vi "Create control.vi"() -> ()   [LabVIEW 2013]
uses:
  Controls/_ui_tools_font.ctl
  Controls/BX.Orientation__LCR _Modified.ctl
  Typedefs/TypeDef_Action.ctl
  <vilib>/Utility/miscctls.llb/LVPointTypeDef.ctl
  Control.lvclass
  <vilib>/Palette API/Palette Menu/Public Type Define/Palette type.ctl
  <vilib>/Palette API/Palette Menu/Public Type Define/Item.ctl
  Engine/Move Speed.ctl
  <userlib>/_OpenG.lib/array/array.llb/Conditional Auto-Indexing Tunnel (String)__ogtk.vi
  <userlib>/_OpenG.lib/file/file.llb/File Exists - Scalar__ogtk.vi
  <userlib>/_OpenG.lib/file/file.llb/Strip Path - Traditional__ogtk.vi
  <userlib>/_OpenG.lib/file/file.llb/Strip Path Extension - String__ogtk.vi
  <userlib>/_OpenG.lib/string/string.llb/To Proper Case (String)__ogtk.vi
  <vilib>/Utility/config.llb/Read Key (String).vi
  <vilib>/Utility/config.llb/Write Key (String).vi
  Fading/SetTransparency(U8).vi
  Fading/_Fade In(I32).vi
  Fading/_Fade Out(I32).vi
  <vilib>/Utility/config.llb/Read Key (Boolean).vi
  <userlib>/_OpenG.lib/file/file.llb/Build Path - Traditional__ogtk.vi
  <vilib>/Utility/config.llb/NI_LVConfig.lvlib
  <vilib>/Palette API/Palette Menu/Palette Menu.lvlib
panel:
  in  "Same decal True/False":bool
  in  "Tab Control":enum32{"False", "True"}(tab)
  in  "Available Icons":picture[][](array[picture])
  in  "Source directory":path
  in  "Icon source":path
  in  "Toolbar 3":cluster{"Font":T1}={"Font"={"Font Name:"="Tahoma", "Size"=13, "Strikeout?"=FALSE, "Italic?"=FALSE, "Underline?"=FALSE, "Outline?"=FALSE, "Shadow?"=FALSE, "Bold?"=TRUE}}
  in  "Add to Project":bool
  in  "Projects":u16(ring) items=["UI Tools.lvproj"]
  in  "Save *.ctl to disk":bool
  in  "Palette":path=path "_LavaCR/CustomControls" caption="<user.lib>\\"
  in  "Front Panels":u16(ring)
  in  "Drop on Front Panel":bool
  in  "Add a copy to UI Tools Palette":bool
  in  "Cancel":bool
  in  "Create":bool
  in  "TRUE Text":string
  in  "Zoom Min":bool
  in  "Zoom Max":bool
  in  "Scale Icon":dbl(slide)=1.0 min=0.5 max=2.0 scale=0.5..2.0 scale format="%.2g"
  in  "Save for version":u16(ring) items=["13.0", "12.0", "11.0", "10.0", "9.0", "8.6", "8.5", "8.2", "8.0"]
  in  "Action":T2=4 items=["Switch when pressed", "Switch when released", "Switch until release", "Latch when pressed", "Latch when released", "Latch until released"]
  in  "Orientations":T3=14
  in  "Button Style":u16(ring)
  in  "Text Color":u32(colorbox)
  in  "FALSE Text":string
  out "PREVIEW":picture
  # "FONT"
  # "FONT"
  # "Preview"
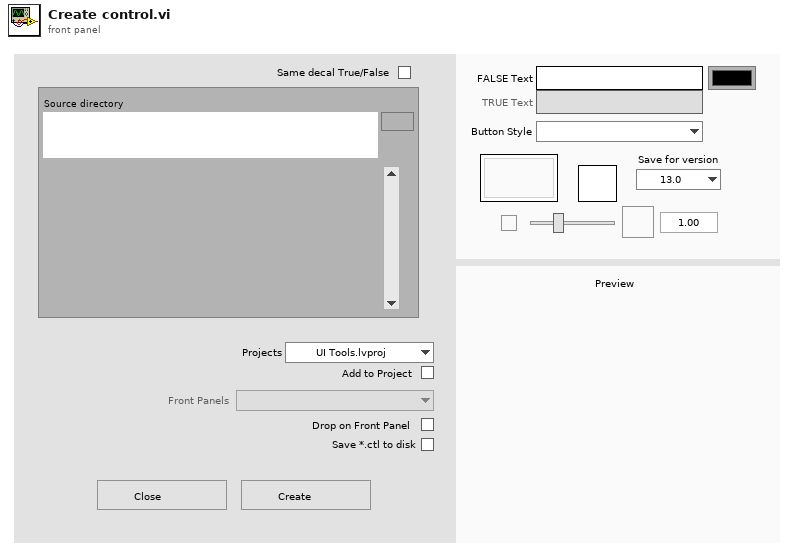
[diagram p1: front panel]
types:
  T1 = typedef "Control.lvclass/_ui_tools_font.ctl" = cluster{"Font Name:":string, "Size":i16, "Strikeout?":bool, "Italic?":bool, "Underline?":bool, "Outline?":bool, "Shadow?":bool, "Bold?":bool}
  T2 = typedef "Control.lvclass/TypeDef_Action.ctl" = u16
  T3 = typedef "Control.lvclass/BX.Orientation__LCR _Modified.ctl" = u8
  T4 = typedef "LVPointTypeDef.ctl" = cluster{"Horizontal":i16, "Vertical":i16}
  T5 = cluster{"Action":refnum<user-event>, "Orientations":refnum<user-event>, "Icon (*.png)":refnum<user-event>, "Font":refnum<user-event>, "Control Text":refnum<user-event>, "Style":refnum<user-event>, "Text Color":refnum<user-event>, "Scale Icon":refnum<user-event>}
  T6 = cluster{"Event Registration Refnum":refnum<event-registration>, "Event Registration Refnum":refnum<event-registration>}
  T7 = typedef "Move Speed.ctl" = enum16{"Normal", "Fast", "Slow", "Instantaneous"}
  T8 = typedef "LVRectTypeDef.ctl" = cluster{"Left":i16, "Top":i16, "Right":i16, "Bottom":i16}
  T9 = cluster{"left":i16, "top":i16, "right":i16, "bottom":i16}
  T10 = cluster{"left":i16, "top":i16, "right":i16, "bottom":i16}[]
  T11 = typedef "LVBoundsTypeDef.ctl" = cluster{"Width":u32, "Height":u32}
  T12 = enum32{"invalid app kind", "Development System", "Run Time System", "Student Edition", "Embedded LabVIEW", "Evaluation", "Custom"}
  T13 = enum32{"Invalid", "Standard", "Closed", "Hidden", "Minimized", "Maximized"}
  T14 = enum32{"Bad", "Idle", "Run top level", "Running"}
  T15 = typedef "Palette Menu.lvlib/Item.ctl" = cluster{"item path":path, "library path (.lvlib)":path, "use default lvlib palette":bool, "short name":string, "place VI contents":bool, "hide synchronized item":bool, "reserve spot for synch item":bool, "configure when placing VI contents":bool}
  T16 = typedef "LVPoint32TypeDef.ctl" = cluster{"Horizontal":i32, "Vertical":i32}
  T17 = typedef "LVPositionTypeDef.ctl" = cluster{"Left":i32, "Top":i32}
  T18 = cluster{"Width":u16, "Style":enum32{"Solid", "Dash", "Dot", "DashDot", "DashDotDot"}}
  T19 = typedef "imagedata.ctl" = cluster{"image type":i32, "image depth":i32, "image":u8[], "mask":u8[], "colors":u32[], "Rectangle":cluster{"left":i16, "top":i16, "right":i16, "bottom":i16}}
  T20 = cluster{"Core":cluster{"Current VI Reference":refnum<vi>, "Close Panel on Exit?":bool, "NI.LV.Dialog namespace":bool, "Menu Launch:App":refnum<vi>, "Local App":refnum<vi>}, "Control":refnum<class "Control.lvclass">, "Errors":cluster{"code":i32, "Short":string, "Long":string, "Critical":bool}[], "user events":cluster{"Action":refnum<user-event>, "Orientations":refnum<user-event>, "Icon (*.png)":refnum<user-event>, "Font":refnum<user-event>, "Control Text":refnum<user-event>, "Style":refnum<user-event>, "Text Color":refnum<user-event>, "Scale Icon":refnum<user-event>}, "last state":cluster{"Action":T2, "Orientations":T3, "Icon (*.png)":path, "Control Text":string, "Style":u16, "Text Color":u32, "Scale":dbl, "Close afterwards":bool}, "config":cluster{"fade":i32, "droplabel":bool}, "file in tmp dir":path, "drop pos":T4}
  T21 = cluster{"code":i32, "Short":string, "Long":string, "Critical":bool}[]
  T22 = cluster{"Action":T2, "Orientations":T3, "Icon (*.png)":path, "Control Text":string, "Style":u16, "Text Color":u32, "Scale":dbl, "Close afterwards":bool}
  T23 = cluster{"Current VI Reference":refnum<vi>, "Close Panel on Exit?":bool, "NI.LV.Dialog namespace":bool, "Menu Launch:App":refnum<vi>, "Local App":refnum<vi>}
  T24 = typedef "NI_LVConfig.lvlib/Config Data RefNum.ctl" = refnum<k1>
  T25 = cluster{"code":i32, "Short":string, "Long":string, "Critical":bool}
  T26 = typedef "Palette Menu.lvlib/Palette type.ctl" = i32
  T27 = typedef "Palette Menu.lvlib/Palette Data.ctl" = cluster{"display name":string, "view format":T28, "palette width":i16, "items":T29, "256 color icon":picture, "B&W color icon":picture, "help information":T30, "palette description":string, "synchronize information":T31}
  T28 = typedef "Palette Menu.lvlib/View Format.ctl" = u16
  T29 = typedef "Palette Menu.lvlib/Items.ctl" = T15[]
  T30 = typedef "Palette Menu.lvlib/Help Info.ctl" = cluster{"help tag":string, "help file path ":path}
  T31 = typedef "Palette Menu.lvlib/Synchronize Info.ctl" = cluster{"synchronize with directory":bool, "synchronize directory path":path}
  T32 = typedef "Control.lvclass/TypeDef_Styles.ctl" = u16
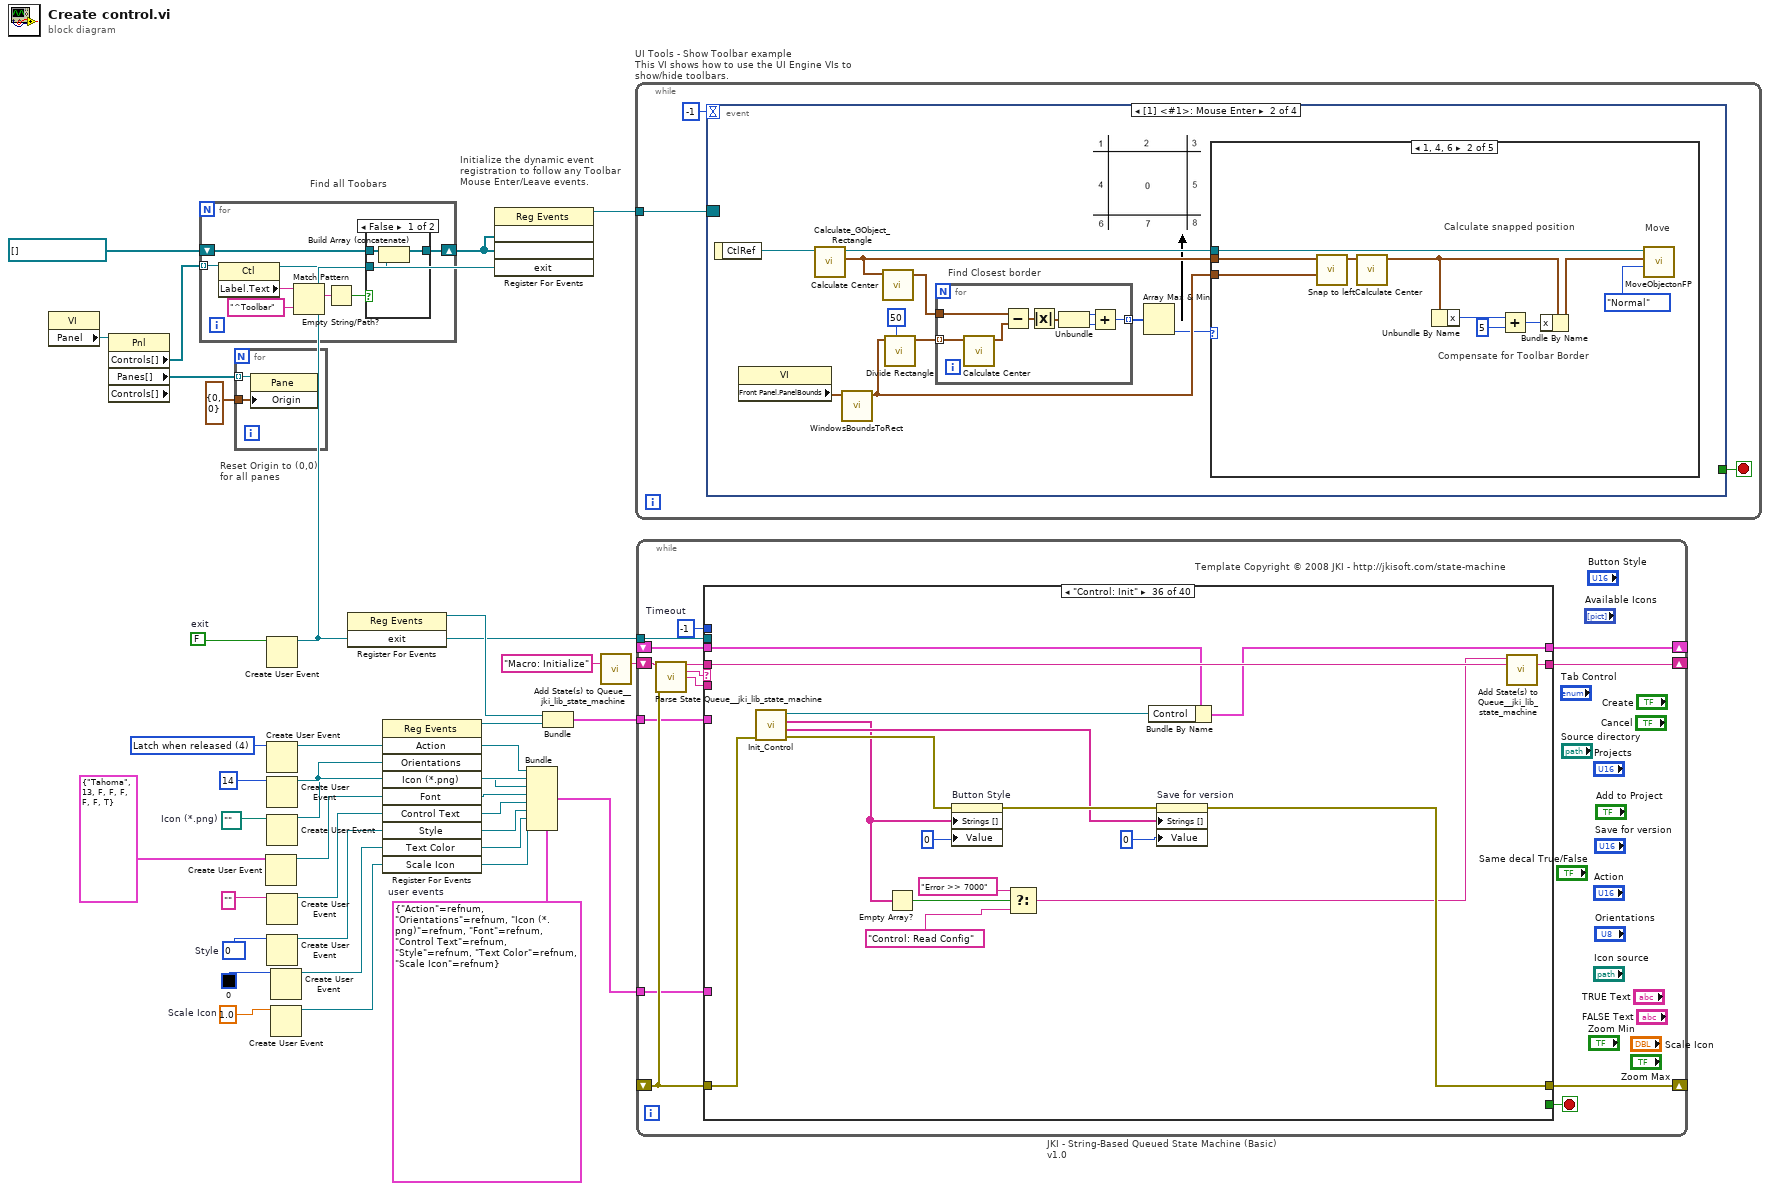
[diagram p0: block diagram]
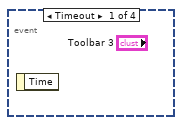
[diagram p3: hidden frame]
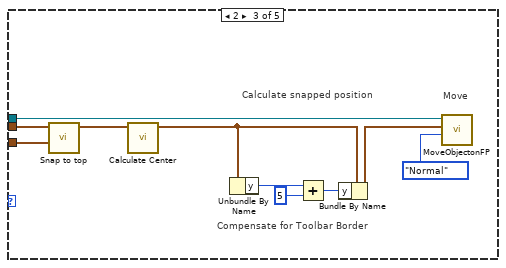
[diagram p5: hidden frame]
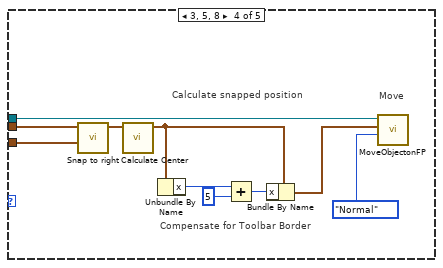
[diagram p6: hidden frame]
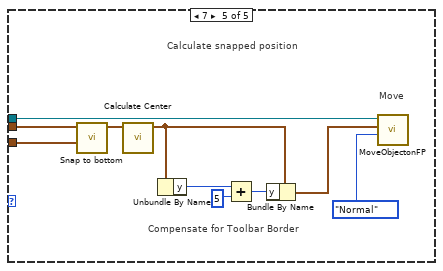
[diagram p7: hidden frame]
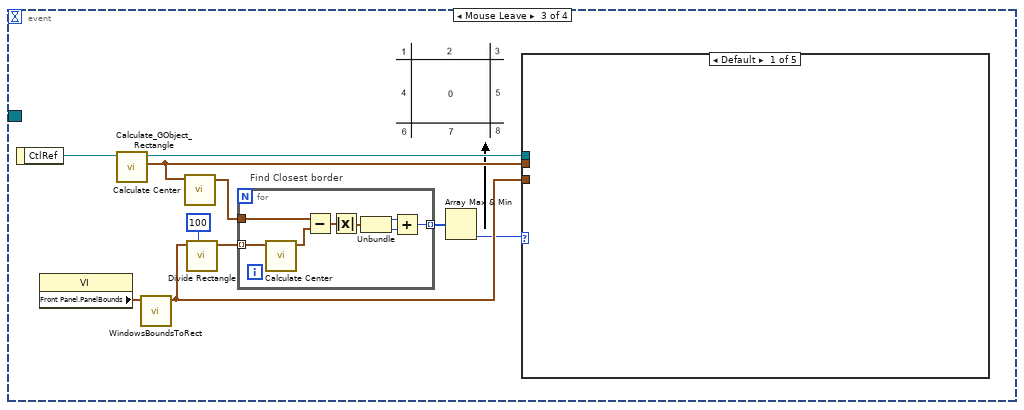
[diagram p8: hidden frame]
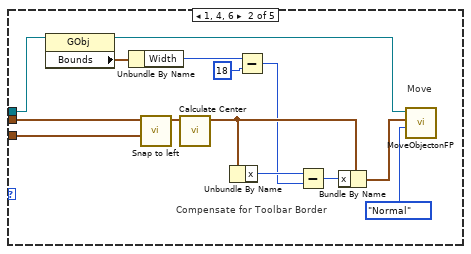
[diagram p9: hidden frame]
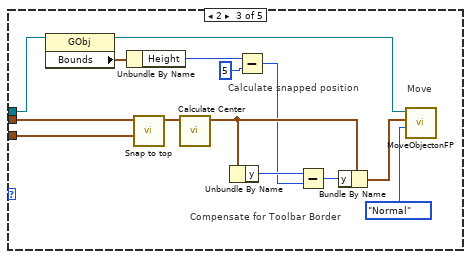
[diagram p10: hidden frame]
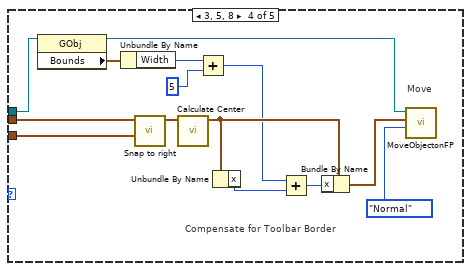
[diagram p11: hidden frame]
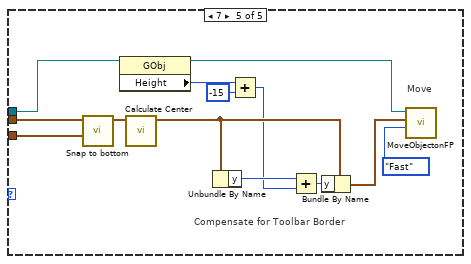
[diagram p12: hidden frame]
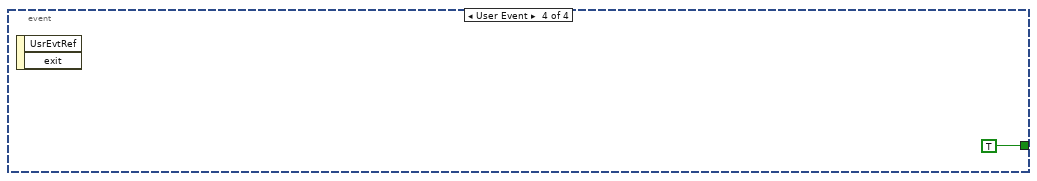
[diagram p13: hidden frame]
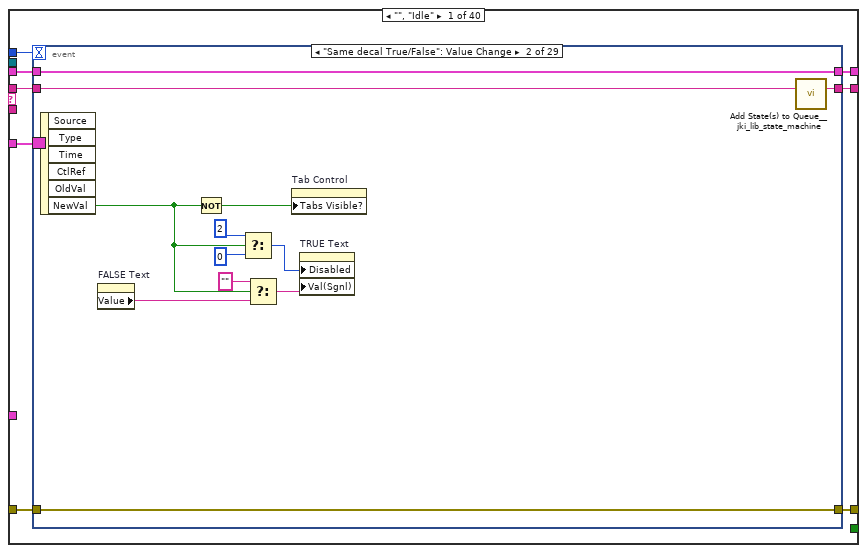
[diagram p14: hidden frame]
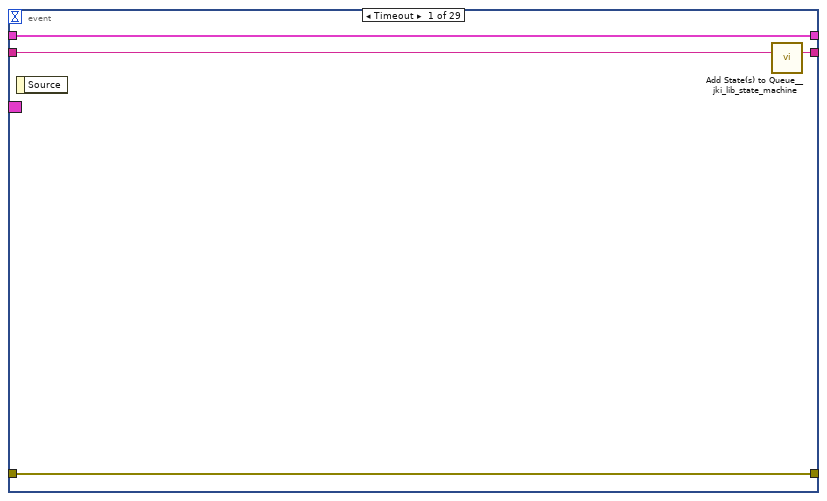
[diagram p15: hidden frame]
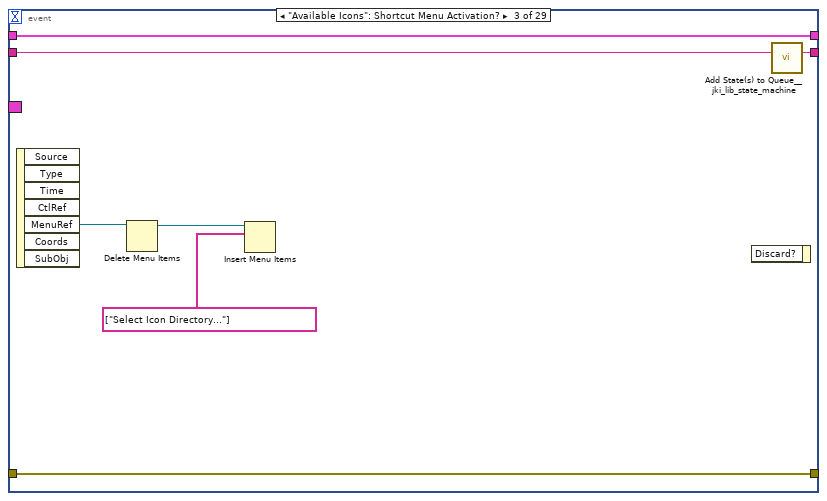
[diagram p16: hidden frame]
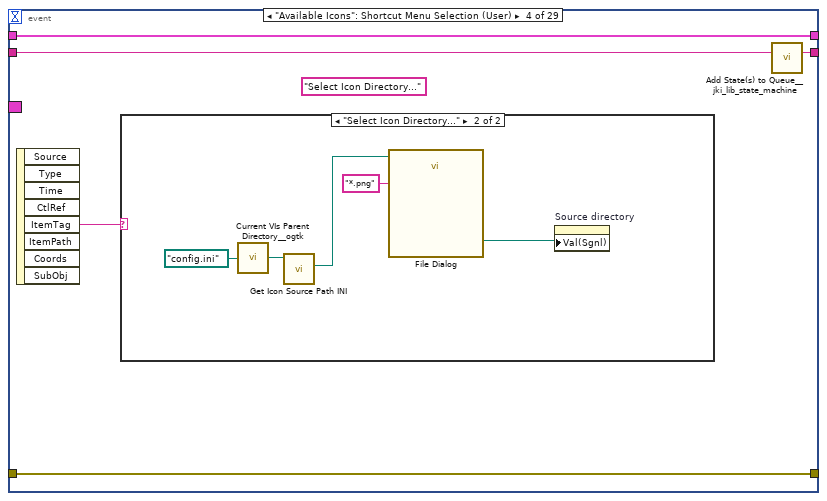
[diagram p17: hidden frame]
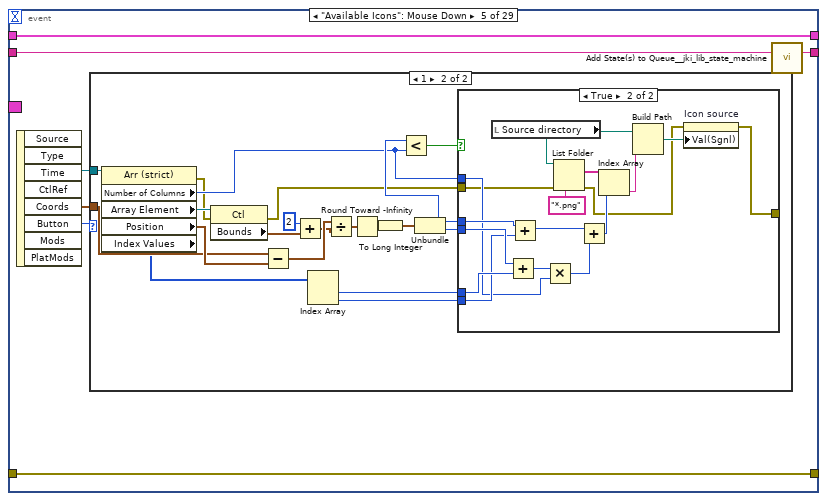
[diagram p19: hidden frame]
diagram:
  w5 = FALSE  # exit
  w13 = T5 {"Action"=refnum, "Orientations"=refnum, "Icon (*.png)"=refnum, "Font"=refnum, "Control Text"=refnum, "Style"=refnum, "Text Color"=refnum, "Scale Icon"=refnum}  # user events
  w18 = 1.0  # Scale Icon
  w22 = u16 0 items=[""]  # Style
  w28 = path ""  # Icon (*.png)
  w32 = T2 4 items=["Switch when pressed", "Switch when released", "Switch until release", "Latch when pressed", "Latch when released", "Latch until released"] ("Action")
  # "Reset Origin to (0,0)\nfor all panes"
  # "Find all Toobars"
  # "Initialize the dynamic event\nregistration to follow any Toolbar\nMouse Enter/Leave events."
  n1 = property class="VI"() -> ("Panel"=w11:refnum<vi>)  [unwired: 2 in, 2 out]
  n2 = property class="Pnl" props=["Controls[]", "Panes[]", "Controls[]"](reference=w11) -> ("Controls[]"=w6:refnum<vi>[], "Panes[]"=w10:refnum<vi>[])  [unwired: 1 in, 3 out]
  n3 = for {
    tunnel: w6 -> [w40] mode=indexing
    shift-right: [w34] -> w7
    shift-left: refnum<vi>[] [] -> [w35]
    n4 = property class="Ctl"(reference=w40) -> (reference out=w33:refnum<vi>, "Label.Text"=w39:string)  [unwired: 1 in, 1 out]
    n5 = Match Pattern(string=w39, regular expression="^Toolbar") -> (match substring=w37:string)  [unwired: 4 out]
    n6 = Empty String/Path?(string/path=w37) -> (empty?=w36:bool)
    n7 = case shown="False" w36 {
      tunnel: [w41 w44] -> w34
      tunnel: w35 -> [w43 w44]
      tunnel: w33 -> [w42 _]
      frame False {
        n8 = Build Array (concatenate)(w43, w42) -> (w41:refnum<vi>[])
      }
      frame True {
      }
    }
  }
  n9 = for {
    tunnel: w10 -> [w46] mode=indexing
    tunnel: T4 {"Horizontal"=0, "Vertical"=0} ("Origin") -> [w45]
    n10 = property class="Pane"(reference=w46, "Origin"=w45) -> ()  [unwired: 1 in, 2 out]
  }
  n11 = Create User Event(user event datatype=T1 {"Font Name:"="Tahoma", "Size"=13, "Strikeout?"=FALSE, "Italic?"=FALSE, "Underline?"=FALSE, "Outline?"=FALSE, "Shadow?"=FALSE, "Bold?"=TRUE} ("Font")) -> (user event=w25:refnum<user-event>)  [unwired: 1 in, 1 out]
  n12 = Create User Event(user event datatype=w5) -> (user event=w1:refnum<user-event>)  [unwired: 1 in, 1 out]
  n13 = Create User Event(user event datatype=w32) -> (user event=w31:refnum<user-event>)  [unwired: 1 in, 1 out]
  n14 = Create User Event(user event datatype=T3 14 ("Orientations")) -> (user event=w30:refnum<user-event>)  [unwired: 1 in, 1 out]
  n15 = Create User Event(user event datatype=w28) -> (user event=w27:refnum<user-event>)  [unwired: 1 in, 1 out]
  n16 = Create User Event(user event datatype="" ("Control Text")) -> (user event=w23:refnum<user-event>)  [unwired: 1 in, 1 out]
  n17 = Create User Event(user event datatype=w22) -> (user event=w21:refnum<user-event>)  [unwired: 1 in, 1 out]
  n18 = Create User Event(user event datatype=u32 0 ("Text Color")) -> (user event=w19:refnum<user-event>)  [unwired: 1 in, 1 out]
  n19 = Create User Event(user event datatype=w18) -> (user event=w17:refnum<user-event>)  [unwired: 1 in, 1 out]
  n20 = register-events(w1) -> (reference out=w4:refnum<event-registration>)  [unwired: 2 in, 1 out]
  n21 = register-events(w31, w30, w27, w25, w23, w21, w19, w17) -> (reference out=w3:refnum<event-registration>)  [unwired: 2 in, 1 out]
  n22 = register-events(w7, w7, w1) -> (reference out=w12:refnum<event-registration>)  [unwired: 2 in, 1 out]
  n23 = Bundle(cluster=w13, "Action"=w31, "Orientations"=w30, "Icon (*.png)"=w27, "Font"=w25, "Control Text"=w23, "Style"=w21, "Text Color"=w19, "Scale Icon"=w17) -> (w14:T5)
  n24 = Bundle("Event Registration Refnum"=w4, "Event Registration Refnum"=w3) -> (w2:T6)  [unwired: 1 out]
  n25 = call <vilib>:"Add State(s) to Queue__jki_lib_state_machine.vi"("State(s) in (\"\")"="Macro: Initialize") -> ("States Out"=w16:string)  [unwired: 2 in, 12 out]
  n26 = while "UI Tools - Show Toolbar example\nThis VI shows how to use the UI Engine VIs to show/hide toolbars." {
    tunnel: w12 -> [w47]
    stop <- w48 stop-if-true
    n27 = event shown="[1] <#1>: Mouse Enter" {
      selector: w47 -> [_ _ _ _]
      dyn-events: _ -> [_ _ _ _]
      timeout: -1 -> [_ _ _ _]
      tunnel: [_ _ _ TRUE ("Discard?")] -> w48
      event Timeout {
        n28 = event-data() -> ()  [unwired: 2 out]
      }
      event Mouse Enter {
        # "Find Closest border"
        n29 = event-data() -> ("CtlRef"=w59:refnum<vi>)  [unwired: 1 out]
        n30 = property class="VI"() -> ("Front Panel.PanelBounds"=w50:T8)  [unwired: 2 in, 2 out]
        n31 = call "Calculate_GObject_Rectangle.vi"("GObject ref"=w59) -> ("Rectangle"=w56:T9, "GObject ref dup"=w51:refnum<vi>)  [unwired: 1 in, 8 out]
        n32 = call "WindowsBoundsToRect.vi"("Windows Bounds"=w50) -> ("Rectangle"=w58:T9)  [unwired: 10 out]
        n33 = call "Calculate Center.vi"("Rectangle"=w56) -> ("Center"=w54:cluster{"x":i32, "y":i32})  [unwired: 10 out]
        n34 = call "Divide Rectangle.vi"("Band (50)"=i16 50, "Rectangle"=w58) -> ("Zones Rectangles"=w55:T10)  [unwired: 1 in, 8 out]
        n35 = for {
          tunnel: w55 -> [w67] mode=indexing
          tunnel: w54 -> [w66]
          tunnel: [w60] -> w53 mode=indexing
          n36 = call "Calculate Center.vi"("Rectangle"=w67) -> ("Center"=w65:cluster{"x":i32, "y":i32})  [unwired: 10 out]
          n37 = Subtract(x=w66, y=w65) -> (x-y=w64:cluster{"x":i32, "y":i32})
          n38 = Absolute Value(x=w64) -> (abs(x)=w63:cluster{"x":i32, "y":i32})
          n39 = Unbundle(w63) -> ("x"=w62:i32, "y"=w61:i32)
          n40 = Add(x=w62, y=w61) -> (x+y=w60:i32)
        }
        n41 = Array Max & Min(array=w53) -> (min index (indices)=w52:i32)  [unwired: 3 out]
        n42 = case shown="1, 4, 6" w52 {
          tunnel: w51 -> [_ w68 w81 w96 w101]
          tunnel: w58 -> [_ w75 w79 w94 w103]
          tunnel: w56 -> [_ w74 w80 w95 w104]
          frame Default {
          }
          frame 1, 4, 6 {
            # "Compensate for Toolbar Border"
            # "Move"
            # "Calculate snapped position"
            n43 = call "Snap to left.vi"("Fixed Rect"=w75, "Rect"=w74) -> ("Snapped to left"=w76:T9)  [unwired: 1 in, 8 out]
            n44 = call "Calculate Center.vi"("Rectangle"=w76) -> ("Center"=w70:cluster{"x":i32, "y":i32})  [unwired: 10 out]
            n45 = Unbundle By Name(w70) -> ("x"=w73:i32)
            n46 = Add(x=w73, y=5) -> (x+y=w71:i32)
            n47 = Bundle By Name(cluster=w70, "x"=w71) -> (w69:cluster{"x":i32, "y":i32})
            n48 = call "MoveObjectonFP.vi"("Move Speed (Instantaneous)"=Move_Speed."Normal", "Center Position for Object"=w69, "GObject"=w68) -> ()  [unwired: 3 in, 6 out]
          }
          frame 2 {
            # "Compensate for Toolbar Border"
            # "Move"
            # "Calculate snapped position"
            n49 = call "Snap to top.vi"("Fixed Rect"=w79, "Rect"=w80) -> ("Snapped to top"=w78:T9)  [unwired: 1 in, 8 out]
            n50 = call "Calculate Center.vi"("Rectangle"=w78) -> ("Center"=w83:cluster{"x":i32, "y":i32})  [unwired: 10 out]
            n51 = Unbundle By Name(w83) -> ("y"=w86:i32)
            n52 = Add(x=w86, y=5) -> (x+y=w84:i32)
            n53 = Bundle By Name(cluster=w83, "y"=w84) -> (w82:cluster{"x":i32, "y":i32})
            n54 = call "MoveObjectonFP.vi"("Move Speed (Instantaneous)"=Move_Speed."Normal", "Center Position for Object"=w82, "GObject"=w81) -> ()  [unwired: 3 in, 6 out]
          }
          frame 3, 5, 8 {
            # "Compensate for Toolbar Border"
            # "Move"
            # "Calculate snapped position"
            n55 = call "Snap to right.vi"("Fixed Rect"=w94, "Rect"=w95) -> ("Snapped to right"=w93:T9)  [unwired: 1 in, 8 out]
            n56 = call "Calculate Center.vi"("Rectangle"=w93) -> ("Center"=w89:cluster{"x":i32, "y":i32})  [unwired: 10 out]
            n57 = Unbundle By Name(w89) -> ("x"=w92:i32)
            n58 = Add(x=w92, y=5) -> (x+y=w90:i32)
            n59 = Bundle By Name(cluster=w89, "x"=w90) -> (w88:cluster{"x":i32, "y":i32})
            n60 = call "MoveObjectonFP.vi"("Move Speed (Instantaneous)"=Move_Speed."Normal", "Center Position for Object"=w88, "GObject"=w96) -> ()  [unwired: 3 in, 6 out]
          }
          frame 7 {
            # "Compensate for Toolbar Border"
            # "Move"
            # "Calculate snapped position"
            n61 = call "Snap to bottom.vi"("Fixed Rect"=w103, "Rect"=w104) -> ("Snapped to bottom"=w102:T9)  [unwired: 1 in, 8 out]
            n62 = call "Calculate Center.vi"("Rectangle"=w102) -> ("Center"=w99:cluster{"x":i32, "y":i32})  [unwired: 10 out]
            n63 = Unbundle By Name(w99) -> ("y"=w106:i32)
            n64 = Add(x=w106, y=5) -> (x+y=w105:i32)
            n65 = Bundle By Name(cluster=w99, "y"=w105) -> (w98:cluster{"x":i32, "y":i32})
            n66 = call "MoveObjectonFP.vi"("Move Speed (Instantaneous)"=Move_Speed."Normal", "Center Position for Object"=w98, "GObject"=w101) -> ()  [unwired: 3 in, 6 out]
          }
        }
      }
      event Mouse Leave {
        # "Find Closest border"
        n67 = event-data() -> ("CtlRef"=w110:refnum<vi>)  [unwired: 1 out]
        n68 = property class="VI"() -> ("Front Panel.PanelBounds"=w109:T8)  [unwired: 2 in, 2 out]
        n69 = call "Calculate_GObject_Rectangle.vi"("GObject ref"=w110) -> ("Rectangle"=w114:T9, "GObject ref dup"=w117:refnum<vi>)  [unwired: 1 in, 8 out]
        n70 = call "WindowsBoundsToRect.vi"("Windows Bounds"=w109) -> ("Rectangle"=w116:T9)  [unwired: 10 out]
        n71 = call "Calculate Center.vi"("Rectangle"=w114) -> ("Center"=w112:cluster{"x":i32, "y":i32})  [unwired: 10 out]
        n72 = call "Divide Rectangle.vi"("Band (50)"=i16 100, "Rectangle"=w116) -> ("Zones Rectangles"=w113:T10)  [unwired: 1 in, 8 out]
        n73 = for {
          tunnel: w113 -> [w125] mode=indexing
          tunnel: w112 -> [w124]
          tunnel: [w118] -> w111 mode=indexing
          n74 = call "Calculate Center.vi"("Rectangle"=w125) -> ("Center"=w123:cluster{"x":i32, "y":i32})  [unwired: 10 out]
          n75 = Subtract(x=w124, y=w123) -> (x-y=w122:cluster{"x":i32, "y":i32})
          n76 = Absolute Value(x=w122) -> (abs(x)=w121:cluster{"x":i32, "y":i32})
          n77 = Unbundle(w121) -> ("x"=w120:i32, "y"=w119:i32)
          n78 = Add(x=w120, y=w119) -> (x+y=w118:i32)
        }
        n79 = Array Max & Min(array=w111) -> (min index (indices)=w108:i32)  [unwired: 3 out]
        n80 = case shown="Default" w108 {
          tunnel: w117 -> [_ w130 w147 w160 w172]
          tunnel: w116 -> [_ w137 w141 w165 w176]
          tunnel: w114 -> [_ w136 w142 w166 w177]
          frame Default {
          }
          frame 1, 4, 6 {
            # "Compensate for Toolbar Border"
            # "Move"
            n81 = property class="GObj"(reference=w130) -> (reference out=w129:refnum<vi>, "Bounds"=w131:T11)  [unwired: 1 in, 1 out]
            n82 = Unbundle By Name(w131) -> ("Width"=w128:u32)
            n83 = call "Snap to left.vi"("Fixed Rect"=w137, "Rect"=w136) -> ("Snapped to left"=w138:T9)  [unwired: 1 in, 8 out]
            n84 = call "Calculate Center.vi"("Rectangle"=w138) -> ("Center"=w133:cluster{"x":i32, "y":i32})  [unwired: 10 out]
            n85 = Unbundle By Name(w133) -> ("x"=w135:i32)
            n86 = Subtract(x=w128, y=u32 18) -> (x-y=w126:u32)
            n87 = Subtract(x=w135, y=w126) -> (x-y=w134:u32)
            n88 = Bundle By Name(cluster=w133, "x"=w134) -> (w132:cluster{"x":i32, "y":i32})
            n89 = call "MoveObjectonFP.vi"("Move Speed (Instantaneous)"=Move_Speed."Normal", "Center Position for Object"=w132, "GObject"=w129) -> ()  [unwired: 3 in, 6 out]
          }
          frame 2 {
            # "Compensate for Toolbar Border"
            # "Move"
            # "Calculate snapped position"
            n90 = property class="GObj"(reference=w147) -> (reference out=w146:refnum<vi>, "Bounds"=w148:T11)  [unwired: 1 in, 1 out]
            n91 = Unbundle By Name(w148) -> ("Height"=w145:u32)
            n92 = call "Snap to top.vi"("Fixed Rect"=w141, "Rect"=w142) -> ("Snapped to top"=w140:T9)  [unwired: 1 in, 8 out]
            n93 = call "Calculate Center.vi"("Rectangle"=w140) -> ("Center"=w150:cluster{"x":i32, "y":i32})  [unwired: 10 out]
            n94 = Unbundle By Name(w150) -> ("y"=w152:i32)
            n95 = Subtract(x=w145, y=u32 5) -> (x-y=w143:u32)
            n96 = Subtract(x=w152, y=w143) -> (x-y=w151:u32)
            n97 = Bundle By Name(cluster=w150, "y"=w151) -> (w149:cluster{"x":i32, "y":i32})
            n98 = call "MoveObjectonFP.vi"("Move Speed (Instantaneous)"=Move_Speed."Normal", "Center Position for Object"=w149, "GObject"=w146) -> ()  [unwired: 3 in, 6 out]
          }
          frame 3, 5, 8 {
            # "Compensate for Toolbar Border"
            # "Move"
            n99 = property class="GObj"(reference=w160) -> (reference out=w159:refnum<vi>, "Bounds"=w161:T11)  [unwired: 1 in, 1 out]
            n100 = Unbundle By Name(w161) -> ("Width"=w156:u32)
            n101 = call "Snap to right.vi"("Fixed Rect"=w165, "Rect"=w166) -> ("Snapped to right"=w164:T9)  [unwired: 1 in, 8 out]
            n102 = call "Calculate Center.vi"("Rectangle"=w164) -> ("Center"=w163:cluster{"x":i32, "y":i32})  [unwired: 10 out]
            n103 = Add(x=w156, y=5) -> (x+y=w154:u32)
            n104 = Unbundle By Name(w163) -> ("x"=w158:i32)
            n105 = Add(x=w154, y=w158) -> (x+y=w157:u32)
            n106 = Bundle By Name(cluster=w163, "x"=w157) -> (w162:cluster{"x":i32, "y":i32})
            n107 = call "MoveObjectonFP.vi"("Move Speed (Instantaneous)"=Move_Speed."Normal", "Center Position for Object"=w162, "GObject"=w159) -> ()  [unwired: 3 in, 6 out]
          }
          frame 7 {
            # "Compensate for Toolbar Border"
            # "Move"
            n108 = call "Snap to bottom.vi"("Fixed Rect"=w176, "Rect"=w177) -> ("Snapped to bottom"=w175:T9)  [unwired: 1 in, 8 out]
            n109 = property class="GObj"(reference=w172) -> (reference out=w171:refnum<vi>, "Height"=w174:u32)  [unwired: 1 in, 1 out]
            n110 = call "Calculate Center.vi"("Rectangle"=w175) -> ("Center"=w179:cluster{"x":i32, "y":i32})  [unwired: 10 out]
            n111 = Unbundle By Name(w179) -> ("y"=w169:i32)
            n112 = Add(x=w174, y=-15) -> (x+y=w168:u32)
            n113 = Add(x=w169, y=w168) -> (x+y=w170:u32)
            n114 = Bundle By Name(cluster=w179, "y"=w170) -> (w178:cluster{"x":i32, "y":i32})
            n115 = call "MoveObjectonFP.vi"("Move Speed (Instantaneous)"=Move_Speed."Fast", "Center Position for Object"=w178, "GObject"=w171) -> ()  [unwired: 3 in, 6 out]
          }
        }
      }
      event User Event {
        n116 = event-data() -> ()  [unwired: 3 out]
      }
    }
  }
  n117 = while "JKI - String-Based Queued State Machine (Basic) v1.0" {
    shift-right: [w188] -> _
    shift-left: _ -> [w187]
    shift-right: [w191] -> _
    shift-left: _ -> [w185]
    shift-right: [w190] -> _
    shift-left: w16 -> [w192]
    tunnel: w14 -> [w184]
    tunnel: w2 -> [w183]
    tunnel: w1 -> [w182]
    stop <- w189 stop-if-true
    w186 = -1  # Timeout
    # "Template Copyright © 2008 JKI - http://jkisoft.com/state-machine"
    n118 = call <vilib>:"Parse State Queue__jki_lib_state_machine.vi"("State Queue"=w192, "Error In (no error)"=w185) -> ("Remaining States"=w194:string, "Current State"=w195:string, "Arguments"=w193:string)  [unwired: 11 out]
    n119 = case shown="\"Control: Init\"" w195 {
      selector: w195 -> [_ _ w613 _ _ _ _ _ _ _ _ _ _ _ _ _ _ _ _ _ _ _ _ _ _ _ _ _ _ _ _ _ _ _ _ _ _ _ _ _]
      tunnel: w194 -> [w203 w612 w617 w627 w645 w655 w680 w692 w696 w708 w732 w745 w756 w775 w789 w796 w802 w805 w814 w859 w880 w903 w908 w919 w923 w943 w967 w996 w1036 w1044 w1067 w1117 w1149 w1191 w1211 w1228 w1240 w1292 w1328 w1360]
      tunnel: w193 -> [_ _ _ _ _ _ w678 _ _ _ _ _ _ _ w785 _ _ w806 w816 _ _ _ _ _ _ _ _ _ _ _ _ _ _ _ _ _ _ _ _ _]
      tunnel: w187 -> [w201 w609 w615 w624 w636 w652 w677 w690 w693 _ w728 w742 w748 w759 w787 w794 w803 w809 w818 w845 w867 w900 w905 w911 w920 w941 w952 w981 w1033 w1041 w1065 w1099 w1147 w1151 w1208 w1226 w1241 w1290 w1335 w1347]
      tunnel: [w200 w610 w619 w625 w642 errorcluster {"status"=FALSE, "code"=0, "source"=""} ("error out") w674 w689 w694 w705 w718 w743 w746 w761 w780 w790 w797 w807 w819 w857 w878 w901 w906 w909 w921 w928 w944 w994 w1034 w1042 w1049 w1107 w1139 w1164 w1209 w1218 w1246 w1294 w1315 w1341] -> w191
      tunnel: w185 -> [w199 w610 w618 w625 w642 w647 _ w689 w694 w705 w729 w743 w746 w762 w781 w791 w798 w808 w820 w857 w878 w901 w906 w909 w921 w931 w947 w994 w1034 w1042 w1048 w1106 w1140 w1169 w1209 w1219 w1247 w1295 w1314 w1342]
      tunnel: [w202 w611 w616 w626 w644 w654 w679 w691 w695 w707 w731 w744 w755 w774 w788 w795 w801 w804 w815 w858 w879 w902 w907 w918 w922 w942 w966 w995 w1035 w1043 w1066 w1116 w1148 w1190 w1210 w1227 w1244 w1293 w1326 w1359] -> w190
      tunnel: [_ _ _ _ _ _ _ TRUE _ _ _ _ _ _ _ _ _ _ _ _ _ _ _ _ _ _ _ _ _ _ _ _ _ _ _ _ _ _ _ _] -> w189
      tunnel: [w198 w609 w615 w624 w643 w652 w677 w690 w693 w706 w728 w742 w748 w758 w787 w794 w803 w809 w818 w845 w867 w900 w905 w911 w920 w941 w951 w980 w1032 w1040 w1064 w1115 w1146 w1189 w1207 w1225 w1237 w1291 w1335 w1346] -> w188
      tunnel: w186 -> [w197 _ _ _ _ _ _ _ _ _ _ _ _ _ _ _ _ _ _ _ _ _ _ _ _ _ _ _ _ _ _ _ _ _ _ _ _ _ _ _]
      tunnel: w184 -> [_ _ _ _ _ _ _ _ _ w701 _ _ _ _ _ _ _ _ _ _ _ _ _ _ _ _ _ _ _ _ _ _ _ _ _ _ _ _ _ _]
      tunnel: w183 -> [w196 _ _ _ _ _ _ _ _ _ w711 _ _ _ _ _ _ _ _ _ _ _ _ _ _ _ _ _ _ _ _ _ _ _ _ _ _ _ _ _]
      tunnel: w182 -> [_ _ _ _ _ _ _ w687 _ _ _ _ _ _ _ _ _ _ _ _ _ _ _ _ _ _ _ _ _ _ _ _ _ _ _ _ _ _ _ _]
      frame "", "Idle" {
        # "executes when the state queue is empty"
        n120 = event shown="[1] \"Same decal True/False\": Value Change" {
          selector: w196 -> [_ _ _ _ _ _ _ _ _ _ _ _ _ _ _ _ _ _ _ _ _ _ _ _ _ _ _ _ _]
          dyn-events: _ -> [_ _ _ _ _ _ _ _ _ _ _ _ _ _ _ _ _ _ _ _ _ _ _ _ _ _ _ _ _]
          timeout: w197 -> [_ _ _ _ _ _ _ _ _ _ _ _ _ _ _ _ _ _ _ _ _ _ _ _ _ _ _ _ _]
          tunnel: w203 -> [w207 w219 w226 w231 w243 w314 w323 w359 w365 w376 w386 w396 w409 w419 w429 w439 w451 w473 w497 w508 w518 w528 w541 w551 w561 w582 w592 w602 w604]
          tunnel: [w206 w218 w225 w230 w242 w313 w322 w358 w364 w375 w385 w395 w408 w418 w428 w438 w450 w472 w496 w507 w517 w527 w540 w550 w560 w581 w591 w601 w603] -> w202
          tunnel: w201 -> [w204 w216 w223 w228 w240 w311 w350 w356 w362 w373 w383 w393 w406 w416 w426 w436 w448 w470 w494 w505 w515 w525 w538 w548 w558 w579 w589 w599 w607]
          tunnel: [w205 w217 w224 w229 w241 w312 w351 w357 w363 w367 w377 w387 w401 w410 w420 w430 w440 w463 w491 w502 w512 w522 w535 w545 w555 w570 w583 w593 w608] -> w200
          tunnel: w199 -> [w205 w217 w224 w229 w241 w312 w351 w357 w363 w368 w378 w388 w402 w411 w421 w431 w441 w462 w487 w499 w510 w520 w533 w543 w553 w572 w584 w594 w608]
          tunnel: [w204 w216 w223 w228 w240 w311 w350 w356 w362 w372 w382 w392 w405 w415 w425 w435 w447 w469 w493 w504 w514 w524 w537 w547 w557 w578 w588 w598 w607] -> w198
          event Timeout {
            n121 = event-data() -> ()  [unwired: 2 out]
            n122 = call <vilib>:"Add State(s) to Queue__jki_lib_state_machine.vi"("State(s) in (\"\")"=w207) -> ("States Out"=w206:string)  [unwired: 2 in, 12 out]
          }
          event "Same decal True/False": Value Change {
            n123 = event-data() -> ("NewVal"=w210:bool)  [unwired: 6 out]
            n124 = property on="FALSE Text" class="Str"() -> ("Value"=w209:string)  [unwired: 2 in, 2 out]
            n125 = Not(x=w210) -> (.not. x?=w215:bool)
            n126 = Select(t=u8 2 ("Disabled"), s=w210, f=u8 0 ("Disabled")) -> (s? t:f=w212:u8)
            n127 = Select(t="", s=w210, f=w209) -> (s? t:f=w211:string)
            n128 = property on="Tab Control" class="TabCtl (strict)"("Tabs Visible?"=w215) -> ()  [unwired: 2 in, 2 out]
            n129 = property on="TRUE Text" class="Str"("Disabled"=w212, "Val(Sgnl)"=w211) -> ()  [unwired: 2 in, 2 out]
            n130 = call <vilib>:"Add State(s) to Queue__jki_lib_state_machine.vi"("State(s) in (\"\")"=w219) -> ("States Out"=w218:string)  [unwired: 2 in, 12 out]
          }
          event "Available Icons": Shortcut Menu Activation? {
            n131 = event-data() -> ("MenuRef"=w222:refnum<k9>)  [unwired: 7 out]
            n132 = Delete Menu Items(9:w222) -> (3:w221:refnum<k9>)  [unwired: 1 in, 3 out]
            n133 = Insert Menu Items(8:string[] ["Select Icon Directory..."] ("item names"), 9:w221) -> ()  [unwired: 1 in, 6 out]
            n134 = event-data() -> ()  [unwired: 1 in, 2 out]
            n135 = call <vilib>:"Add State(s) to Queue__jki_lib_state_machine.vi"("State(s) in (\"\")"=w226) -> ("States Out"=w225:string)  [unwired: 2 in, 12 out]
          }
          event "Available Icons": Shortcut Menu Selection (User) {
            (unwired) "Select Icon Directory..."
            n136 = event-data() -> ("ItemTag"=w227:string)  [unwired: 8 out]
            n137 = case shown="\"Select Icon Directory...\"" w227 {
              frame "False", Default {
              }
              frame "Select Icon Directory..." {
                n138 = call <userlib>:"Current VIs Parent Directory__ogtk.vi"("Relative path (.)"=path "config.ini") -> ("Parent Directory (+ Relative)"=w234:path)  [unwired: 4 out]
                n139 = call "Get Icon Source Path INI.vi"("config.ini path"=w234) -> ("Icon source dir"=w232:path)  [unwired: 2 in, 8 out]
                n140 = call "File Dialog"("start path"=w232, "pattern (all files)"="*.png") -> ("selected path"=w233:path)  [unwired: 5 in, 8 out]
                n141 = property on="Source directory" class="Path"("Val(Sgnl)"=w233) -> ()  [unwired: 2 in, 2 out]
              }
            }
            n142 = call <vilib>:"Add State(s) to Queue__jki_lib_state_machine.vi"("State(s) in (\"\")"=w231) -> ("States Out"=w230:string)  [unwired: 2 in, 12 out]
          }
          event "Available Icons": Mouse Down {
            n143 = event-data() -> ("CtlRef"=w239:refnum<vi>, "Coords"=w238:T16, "Button"=w237:u16)  [unwired: 6 out]
            n144 = case shown="1" w237 {
              tunnel: w239 -> [_ w263]
              tunnel: w238 -> [_ w260]
              frame Default {
              }
              frame 1 {
                n145 = property class="Arr (strict)"(reference=w263) -> (error out=w245:errorcluster, "Number of Columns"=w246:u32, "Array Element"=w262:refnum<vi>, "Position"=w261:T17, "Index Values"=w255:u32[])  [unwired: 1 in, 1 out]
                n146 = property class="Ctl"(reference=w262, error in=w245) -> (error out=w244:errorcluster, "Bounds"=w251:T11)  [unwired: 1 out]
                n147 = Subtract(x=w260, y=w261) -> (x-y=w259:T16)
                n148 = Add(x=2, y=w251) -> (x+y=w250:T11)
                n149 = Index Array(array=w255) -> (element #1=w253:u32, element #2=w252:u32)  [unwired: 2 in]
                n150 = Divide(x=w259, y=w250) -> (x/y=w258:cluster{dbl, dbl})
                n151 = Round Toward -Infinity(1:w258) -> (0:w257:cluster{dbl, dbl})
                n152 = To Long Integer(number=w257) -> (32bit integer=w256:cluster{i32, i32})
                n153 = Unbundle(w256) -> (w247:i32, w254:i32)
                n154 = Less?(x=w247, y=w246) -> (x < y?=w248:bool)
                n155 = case shown="True" w248 {
                  tunnel: w247 -> [_ w280]
                  tunnel: w254 -> [_ w279]
                  tunnel: w253 -> [_ w269]
                  tunnel: w252 -> [_ w268]
                  tunnel: w246 -> [_ w267]
                  tunnel: [_ w265] -> _
                  tunnel: w244 -> [_ w264]
                  frame False {
                  }
                  frame True {
                    n156 = local read "Source directory"() -> (w272:path)
                    n157 = Add(x=w279, y=w269) -> (x+y=w275:u32)
                    n158 = Add(x=w280, y=w268) -> (x+y=w273:u32)
                    n159 = Multiply(x=w275, y=w267) -> (x*y=w274:u32)
                    n160 = List Folder(path=w272, pattern="*.png", error in=w264) -> (filenames=w277:string[], error out=w266:errorcluster)  [unwired: 3 out]
                    n161 = Add(x=w273, y=w274) -> (x+y=w276:u32)
                    n162 = Index Array(array=w277, index=w276) -> (element=w271:string)
                    n163 = Build Path(base path=w272, name or relative path=w271) -> (appended path=w270:path)
                    n164 = property on="Icon source" class="Path"(error in=w266, "Val(Sgnl)"=w270) -> (error out=w265:errorcluster)  [unwired: 1 in, 1 out]
                  }
                }
              }
            }
            n165 = call <vilib>:"Add State(s) to Queue__jki_lib_state_machine.vi"("State(s) in (\"\")"=w243) -> ("States Out"=w242:string)  [unwired: 2 in, 12 out]
          }
          event "Source directory": Value Change {
            w292 = T18 {"Width"=2, "Style"=enum."Dash"} ("pen")
            w288 = i16 4 ("oval width")
            n166 = event-data() -> ("NewVal"=w282:path)  [unwired: 1 out]
            n167 = property on="Icon source" class="Path"() -> ("Value"=w305:path)  [unwired: 2 in, 2 out]
            n168 = Strip Path(path=w305) -> (name=w303:string)  [unwired: 1 out]
            n169 = List Folder(path=w282, pattern="*.png") -> (path out=w309:path, filenames=w304:string[], error out=w283:errorcluster)  [unwired: 1 in, 2 out]
            n170 = property on="Available Icons" class="Arr (strict)"() -> ("Number of Columns"=w294:u32, "Array Element"=w293:refnum<vi>)  [unwired: 2 in, 2 out]
            n171 = Search 1D Array(1D array=w304, element=w303) -> (index of element=w302:i32)  [unwired: 1 out]
            n172 = for {
              tunnel: w304 -> [w318] mode=indexing
              tunnel: w309 -> [w319]
              tunnel: [w315] -> w308 mode=indexing
              tunnel: w283 -> [_]
              n173 = Build Path(base path=w319, name or relative path=w318) -> (appended path=w317:path)
              n174 = call <vilib>:"Read PNG File.vi"("path to PNG file"=w317) -> ("image data"=w316:T19)  [unwired: 1 in, 9 out]
              n175 = call <vilib>:"Draw Flattened Pixmap.vi"("image data"=w316) -> ("new picture"=w315:picture)  [unwired: 1 in, 7 out]
            }
            n176 = property class="Ctl"(reference=w293) -> ("Bounds"=w291:T11)  [unwired: 1 in, 2 out]
            n177 = Unbundle By Name(w292) -> ("Width"=w290:u16)
            n178 = Array Size(array=w308) -> (size(s)=w307:i32)
            n179 = Subtract(x=w291, y=w290) -> (x-y=w289:T11)
            n180 = Quotient & Remainder(x=w302, y=w294) -> (x-y*floor(x/y)=w295:u32, floor(x/y)=w296:u32)
            n181 = Quotient & Remainder(x=w307, y=w294) -> (floor(x/y)=w306:u32)  [unwired: 1 out]
            n182 = Reshape Array(w308, w306, w294) -> (w301:picture[][])
            n183 = Index Array(array=w301, index (row)=w296, index (col)=w295) -> (element=w299:picture)
            n184 = Subtract(x=w289, y=w288) -> (x-y=w287:T11)
            n185 = Unbundle(w287) -> ("Width"=w281:u32, "Height"=w284:u32)
            n186 = Bundle(cluster=T9 {"left"=0, "top"=0, "right"=42, "bottom"=42} ("rect"), "right"=w281, "bottom"=w284) -> (w285:T9)  [unwired: 2 out]
            n187 = call <vilib>:"Draw Round Rect.vi"("picture"=w299, "oval width"=w288, "rect"=w285, "color(black)"=u32 35073, "oval height"=w288, "pen"=w292) -> ("new picture"=w298:picture)  [unwired: 1 in, 2 out]
            n188 = Replace Array Subset(array=w301, new element=w298, index (row)=w296, index (col)=w295) -> (w300:picture[][])
            n189 = property on="Available Icons" class="Arr (strict)"("Value"=w300) -> ()  [unwired: 2 in, 2 out]
            n190 = call <vilib>:"Add State(s) to Queue__jki_lib_state_machine.vi"("State(s) in (\"\")"=w314) -> ("States Out"=w313:string)  [unwired: 2 in, 12 out]
          }
          event "Create": Value Change {
            # "If batch processing needed, prepare for it."
            # "Prepare for the execution list based on\nuser choices."
            n191 = event-data() -> ()  [unwired: 2 out]
            n192 = property on="Add to Project" class="Bool (strict)"() -> ("Value"=w321:bool)  [unwired: 2 in, 2 out]
            n193 = property on="Icon source" class="Path"() -> ("Value"=w320:path)  [unwired: 2 in, 2 out]
            n194 = call-poly <userlib>:"File Exists__ogtk.vi"("file path"=w320) -> ("is directory"=w338:bool, "exists"=w337:bool)  [unwired: 6 in]
            n195 = And(x=w338, y=w337) -> (x .and. y?=w335:bool)
            n196 = Build Array("Save *.ctl to disk", "Add a copy to UI Tools Palette", w321, "Drop on Front Panel") -> (w342:bool[])
            n197 = Build Array("Control: Save Control to Disk", "Control: Add to palette", "Control: Add to Project", "Control: Add to FP") -> (w341:string[])
            n198 = call-poly <userlib>:"Conditional Auto-Indexing Tunnel__ogtk.vi"("Array in"=w341, "Elements to keep"=w342) -> ("Filtered Array out"=w340:string[])  [unwired: 5 out]
            n199 = for {
              tunnel: w340 -> [w354] mode=indexing
              shift-right: [w352] -> w326
              shift-left: "" -> [w353]
              n200 = call <vilib>:"Add State(s) to Queue__jki_lib_state_machine.vi"("State(s) in (\"\")"=w353, "State(s) at Back (\"\")"=w354) -> ("States Out"=w352:string)  [unwired: 1 in, 12 out]
            }
            n201 = Select(t="Control: Prepare batch", s=w335, f="") -> (s? t:f=w329:string)
            n202 = Select(t="Macro: Exit", s=FALSE ("End program afterwards"), f="") -> (s? t:f=w328:string)
            n203 = call <vilib>:"Add State(s) to Queue__jki_lib_state_machine.vi"("State(s) in Front (\"\")"="Control: Save Temp Control", "State(s) in (\"\")"=w326, "State(s) at Back (\"\")"="Control: Save Config\nControl: Delete Temp Control") -> ("States Out"=w330:string)  [unwired: 12 out]
            n204 = call <vilib>:"Add State(s) to Queue__jki_lib_state_machine.vi"("State(s) in Front (\"\")"=w329, "State(s) in (\"\")"=w330, "State(s) at Back (\"\")"=w328) -> ("States Out"=w324:string)  [unwired: 12 out]
            n205 = call <vilib>:"Add State(s) to Queue__jki_lib_state_machine.vi"("State(s) in Front (\"\")"=w324, "State(s) in (\"\")"=w323) -> ("States Out"=w322:string)  [unwired: 1 in, 12 out]
          }
          event "Cancel": Value Change {
            # "Exit Button Value Change (pressed) Event\n(this executes Macro: Exit to terminate the VI)"
            n206 = event-data() -> ()  [unwired: 2 out]
            n207 = call <vilib>:"Add State(s) to Queue__jki_lib_state_machine.vi"("State(s) in Front (\"\")"="Macro: Exit", "State(s) in (\"\")"=w359) -> ("States Out"=w358:string)  [unwired: 1 in, 12 out]
          }
          event Menu Selection (User) {
            # "Menu selections (including rtm file)"
            n208 = event-data() -> ("ItemTag"=w360:string)  [unwired: 7 out]
            n209 = case shown="\"About\"" w360 {
              tunnel: [_ "UI: FadeOut >> 200\nAbout\nUI: FadeIn >> 200"] -> w361
              frame Default {
              }
              frame "About" {
              }
            }
            n210 = call <vilib>:"Add State(s) to Queue__jki_lib_state_machine.vi"("State(s) in Front (\"\")"=w361, "State(s) in (\"\")"=w365) -> ("States Out"=w364:string)  [unwired: 1 in, 12 out]
          }
          event Value Change {
            n211 = event-data() -> ("NewVal"=w369:T1)  [unwired: 6 out]
            n212 = Unbundle By Name(w373) -> ("Control"=w371:refnum<class "Control.lvclass">)
            n213 = call-dynamic "Write Text Font.vi"("error in (no error)"=w368, "Font"=w369, "Control in"=w371) -> ("error out"=w367:errorcluster, "Control out"=w370:refnum<class "Control.lvclass">)  [unwired: 7 out]
            n214 = Bundle By Name(cluster=w373, "Control"=w370) -> (w372:T20)
            n215 = call <vilib>:"Add State(s) to Queue__jki_lib_state_machine.vi"("State(s) in Front (\"\")"="Preview", "State(s) in (\"\")"=w376) -> ("States Out"=w375:string)  [unwired: 1 in, 12 out]
          }
          event "Scale Icon": Value Change {
            n216 = event-data() -> ("NewVal"=w379:dbl)  [unwired: 6 out]
            n217 = Unbundle By Name(w383) -> ("Control"=w381:refnum<class "Control.lvclass">)
            n218 = call-dynamic "Write Scale Icon.vi"("error in (no error)"=w378, "Scale Icon"=w379, "Control in"=w381) -> ("error out"=w377:errorcluster, "Control out"=w380:refnum<class "Control.lvclass">)  [unwired: 7 out]
            n219 = Bundle By Name(cluster=w383, "Control"=w380) -> (w382:T20)
            n220 = call <vilib>:"Add State(s) to Queue__jki_lib_state_machine.vi"("State(s) in Front (\"\")"="Preview", "State(s) in (\"\")"=w386) -> ("States Out"=w385:string)  [unwired: 1 in, 12 out]
          }
          event Value Change {
            n221 = event-data() -> ("NewVal"=w389:T2)  [unwired: 6 out]
            n222 = Unbundle By Name(w393) -> ("Control"=w391:refnum<class "Control.lvclass">)
            n223 = call-dynamic "Write Action.vi"("error in (no error)"=w388, "Action"=w389, "Control in"=w391) -> ("error out"=w387:errorcluster, "Control out"=w390:refnum<class "Control.lvclass">)  [unwired: 7 out]
            n224 = Bundle By Name(cluster=w393, "Control"=w390) -> (w392:T20)
            n225 = call <vilib>:"Add State(s) to Queue__jki_lib_state_machine.vi"("State(s) in Front (\"\")"="Preview", "State(s) in (\"\")"=w396) -> ("States Out"=w395:string)  [unwired: 1 in, 12 out]
          }
          event "FALSE Text", "TRUE Text": Value Change {
            n226 = event-data() -> ()  [unwired: 7 out]
            n227 = Unbundle By Name(w406) -> ("Control"=w404:refnum<class "Control.lvclass">)
            n228 = local read "Same decal True/False"() -> (w399:bool)
            n229 = local read "FALSE Text"() -> (w397:string)
            n230 = local read "TRUE Text"() -> (w398:string)
            n231 = Select(t=w397, s=w399, f=w398) -> (s? t:f=w400:string)
            n232 = call-dynamic "Write Control Text.vi"("error in (no error)"=w402, "True Text"=w400, "False Text"=w397, "Control in"=w404) -> ("error out"=w401:errorcluster, "Control out"=w403:refnum<class "Control.lvclass">)  [unwired: 6 out]
            n233 = Bundle By Name(cluster=w406, "Control"=w403) -> (w405:T20)
            n234 = call <vilib>:"Add State(s) to Queue__jki_lib_state_machine.vi"("State(s) in Front (\"\")"="Preview", "State(s) in (\"\")"=w409) -> ("States Out"=w408:string)  [unwired: 1 in, 12 out]
          }
          event Value Change {
            n235 = event-data() -> ("NewVal"=w412:T3)  [unwired: 6 out]
            n236 = Unbundle By Name(w416) -> ("Control"=w414:refnum<class "Control.lvclass">)
            n237 = call-dynamic "Write Orientations.vi"("error in (no error)"=w411, "Orientations"=w412, "Control in"=w414) -> ("error out"=w410:errorcluster, "Control out"=w413:refnum<class "Control.lvclass">)  [unwired: 7 out]
            n238 = Bundle By Name(cluster=w416, "Control"=w413) -> (w415:T20)
            n239 = call <vilib>:"Add State(s) to Queue__jki_lib_state_machine.vi"("State(s) in Front (\"\")"="Preview", "State(s) in (\"\")"=w419) -> ("States Out"=w418:string)  [unwired: 1 in, 12 out]
          }
          event "Text Color": Value Change {
            n240 = event-data() -> ("NewVal"=w422:u32)  [unwired: 6 out]
            n241 = Unbundle By Name(w426) -> ("Control"=w424:refnum<class "Control.lvclass">)
            n242 = call-dynamic "Write Text Color.vi"("error in (no error)"=w421, "Text Color"=w422, "Control.lvclass in"=w424) -> ("error out"=w420:errorcluster, "Control.lvclass out"=w423:refnum<class "Control.lvclass">)  [unwired: 7 out]
            n243 = Bundle By Name(cluster=w426, "Control"=w423) -> (w425:T20)
            n244 = call <vilib>:"Add State(s) to Queue__jki_lib_state_machine.vi"("State(s) in Front (\"\")"="Preview", "State(s) in (\"\")"=w429) -> ("States Out"=w428:string)  [unwired: 1 in, 12 out]
          }
          event "Button Style": Value Change {
            n245 = event-data() -> ("NewVal"=w432:u16)  [unwired: 6 out]
            n246 = Unbundle By Name(w436) -> ("Control"=w434:refnum<class "Control.lvclass">)
            n247 = call-dynamic "Write Style.vi"("error in (no error)"=w431, "Style index (-1)"=w432, "Control in"=w434) -> ("error out"=w430:errorcluster, "Control out"=w433:refnum<class "Control.lvclass">)  [unwired: 1 in, 6 out]
            n248 = Bundle By Name(cluster=w436, "Control"=w433) -> (w435:T20)
            n249 = call <vilib>:"Add State(s) to Queue__jki_lib_state_machine.vi"("State(s) in Front (\"\")"="Preview", "State(s) in (\"\")"=w439) -> ("States Out"=w438:string)  [unwired: 1 in, 12 out]
          }
          event "Save for version": Value Change {
            n250 = event-data() -> ("NewVal"=w444:u16)  [unwired: 6 out]
            n251 = Unbundle By Name(w448) -> ("Control"=w443:refnum<class "Control.lvclass">)
            n252 = property on="Save for version" class="Ring (strict)"() -> ("Strings []"=w445:string[])  [unwired: 2 in, 2 out]
            n253 = Index Array(array=w445, index=w444) -> (element=w446:string)
            n254 = call-dynamic "Write Save for version.vi"("error in (no error)"=w441, "Save for version"=w446, "Control.lvclass in"=w443) -> ("error out"=w440:errorcluster, "Control.lvclass out"=w442:refnum<class "Control.lvclass">)  [unwired: 7 out]
            n255 = Bundle By Name(cluster=w448, "Control"=w442) -> (w447:T20)
            n256 = call <vilib>:"Add State(s) to Queue__jki_lib_state_machine.vi"("State(s) in Front (\"\")"="Preview", "State(s) in (\"\")"=w451) -> ("States Out"=w450:string)  [unwired: 1 in, 12 out]
          }
          event "Icon source": Value Change {
            # "If batch processing... no addition on FP possible"
            # "TO DO: \n\nif a directory, then prepare for batch processing.\n\nThe control text will be the name of the png icon file.\n\nPreview of the first png icon found in the directories will be shown as preview."
            n257 = event-data() -> ("NewVal"=w460:path)  [unwired: 6 out]
            n258 = call-poly <userlib>:"File Exists__ogtk.vi"("file path"=w460) -> ("is directory"=w459:bool, "exists"=w458:bool)  [unwired: 6 in]
            n259 = And(x=w459, y=w458) -> (x .and. y?=w457:bool)
            n260 = Unbundle By Name(w470) -> ("Control"=w461:refnum<class "Control.lvclass">)
            n261 = call-dynamic "Load Icon.vi"("error in (no error)"=w462, "Icon path False"=w460, "Control in"=w461) -> ("error out"=w465:errorcluster, "Control out"=w466:refnum<class "Control.lvclass">)  [unwired: 1 in, 6 out]
            n262 = call-poly <userlib>:"Strip Path__ogtk.vi"("path"=w460) -> ("stripped path"=w456:path, "name"=w468:string)
            n263 = local read "Same decal True/False"() -> (w455:bool)
            n264 = case shown="True" w457 {
              frame False {
                n265 = property on="Drop on Front Panel" class="Bool (strict)"("Disabled"=u8 0) -> ()  [unwired: 2 in, 2 out]
              }
              frame True {
                n266 = property on="Drop on Front Panel" class="Bool (strict)"("Value"=FALSE ("Drop on Front Panel"), "Disabled"=u8 2) -> ()  [unwired: 2 in, 2 out]
              }
            }
            n267 = call-poly <userlib>:"Strip Path Extension__ogtk.vi"("path"=w468) -> ("root"=w467:string)  [unwired: 1 out]
            n268 = property on="Source directory" class="Path"("Val(Sgnl)"=w456) -> ()  [unwired: 2 in, 2 out]
            n269 = call-poly <userlib>:"To Proper Case__ogtk.vi"("string"=w467) -> ("proper case string"=w454:string)  [unwired: 4 out]
            n270 = local read "TRUE Text"() -> (w452:string)
            n271 = local write "FALSE Text"(w454) -> ()
            n272 = Select(t=w454, s=w455, f=w452) -> (s? t:f=w453:string)
            n273 = call-dynamic "Write Control Text.vi"("error in (no error)"=w465, "True Text"=w453, "False Text"=w454, "Control in"=w466) -> ("error out"=w463:errorcluster, "Control out"=w464:refnum<class "Control.lvclass">)  [unwired: 6 out]
            n274 = Bundle By Name(cluster=w470, "Control"=w464) -> (w469:T20)
            n275 = call <vilib>:"Add State(s) to Queue__jki_lib_state_machine.vi"("State(s) in Front (\"\")"="Preview", "State(s) in (\"\")"=w473) -> ("States Out"=w472:string)  [unwired: 1 in, 12 out]
          }
          event User Event {
            n276 = event-data() -> ("Font Name:"=w477:string, "Size"=w485:i16, "Strikeout?"=w484:bool, "Italic?"=w483:bool, "Underline?"=w482:bool, "Outline?"=w481:bool, "Shadow?"=w480:bool, "Bold?"=w479:bool)  [unwired: 5 out]
            n277 = Unbundle By Name(w494) -> ("Control"=w489:refnum<class "Control.lvclass">)
            n278 = call-dynamic "Read Text Font.vi"("error in (no error)"=w487, "Control in"=w489) -> ("error out"=w488:errorcluster, "Font"=w486:T1, "Control out"=w490:refnum<class "Control.lvclass">)  [unwired: 7 out]
            n279 = Bundle By Name(cluster=w486, "Font Name:"=w477, "Size"=w485, "Strikeout?"=w484, "Italic?"=w483, "Underline?"=w482, "Outline?"=w481, "Shadow?"=w480, "Bold?"=w479) -> (w478:T1)
            n280 = property on="Font" class="Clust (strict)"("Value"=w478) -> ()  [unwired: 2 in, 2 out]
            n281 = call-dynamic "Write Text Font.vi"("error in (no error)"=w488, "Font"=w478, "Control in"=w490) -> ("error out"=w491:errorcluster, "Control out"=w492:refnum<class "Control.lvclass">)  [unwired: 7 out]
            n282 = Bundle By Name(cluster=w494, "Control"=w492) -> (w493:T20)
            n283 = call <vilib>:"Add State(s) to Queue__jki_lib_state_machine.vi"("State(s) in Front (\"\")"="Preview", "State(s) in (\"\")"=w497) -> ("States Out"=w496:string)  [unwired: 1 in, 12 out]
          }
          event User Event {
            n284 = event-data() -> ("Scale Icon"=w500:dbl)  [unwired: 5 out]
            n285 = Unbundle By Name(w505) -> ("Control"=w501:refnum<class "Control.lvclass">)
            n286 = property on="Scale Icon" class="Slide (strict)"(error in=w499, "Value"=w500) -> (error out=w498:errorcluster)  [unwired: 1 in, 1 out]
            n287 = call-dynamic "Write Scale Icon.vi"("error in (no error)"=w498, "Scale Icon"=w500, "Control in"=w501) -> ("error out"=w502:errorcluster, "Control out"=w503:refnum<class "Control.lvclass">)  [unwired: 7 out]
            n288 = Bundle By Name(cluster=w505, "Control"=w503) -> (w504:T20)
            n289 = call <vilib>:"Add State(s) to Queue__jki_lib_state_machine.vi"("State(s) in Front (\"\")"="Preview", "State(s) in (\"\")"=w508) -> ("States Out"=w507:string)  [unwired: 1 in, 12 out]
          }
          event User Event {
            n290 = event-data() -> ("Action"=w509:T2)  [unwired: 5 out]
            n291 = Unbundle By Name(w515) -> ("Control"=w511:refnum<class "Control.lvclass">)
            n292 = property on="Action" class="Ring (strict)"("Value"=w509) -> ()  [unwired: 2 in, 2 out]
            n293 = call-dynamic "Write Action.vi"("error in (no error)"=w510, "Action"=w509, "Control in"=w511) -> ("error out"=w512:errorcluster, "Control out"=w513:refnum<class "Control.lvclass">)  [unwired: 7 out]
            n294 = Bundle By Name(cluster=w515, "Control"=w513) -> (w514:T20)
            n295 = call <vilib>:"Add State(s) to Queue__jki_lib_state_machine.vi"("State(s) in Front (\"\")"="Preview", "State(s) in (\"\")"=w518) -> ("States Out"=w517:string)  [unwired: 1 in, 12 out]
          }
          event User Event {
            n296 = event-data() -> ("Orientations"=w519:T3)  [unwired: 5 out]
            n297 = Unbundle By Name(w525) -> ("Control"=w521:refnum<class "Control.lvclass">)
            n298 = property on="Orientations" class="Ring (strict)"("Value"=w519) -> ()  [unwired: 2 in, 2 out]
            n299 = call-dynamic "Write Orientations.vi"("error in (no error)"=w520, "Orientations"=w519, "Control in"=w521) -> ("error out"=w522:errorcluster, "Control out"=w523:refnum<class "Control.lvclass">)  [unwired: 7 out]
            n300 = Bundle By Name(cluster=w525, "Control"=w523) -> (w524:T20)
            n301 = call <vilib>:"Add State(s) to Queue__jki_lib_state_machine.vi"("State(s) in Front (\"\")"="Preview", "State(s) in (\"\")"=w528) -> ("States Out"=w527:string)  [unwired: 1 in, 12 out]
          }
          event User Event {
            n302 = event-data() -> ("Control Text"=w530:string)  [unwired: 5 out]
            n303 = Unbundle By Name(w538) -> ("Control"=w534:refnum<class "Control.lvclass">)
            n304 = local read "Same decal True/False"() -> (w532:bool)
            n305 = local read "TRUE Text"() -> (w531:string)
            n306 = local write "FALSE Text"(w530) -> ()
            n307 = Select(t=w530, s=w532, f=w531) -> (s? t:f=w529:string)
            n308 = call-dynamic "Write Control Text.vi"("error in (no error)"=w533, "True Text"=w529, "False Text"=w530, "Control in"=w534) -> ("error out"=w535:errorcluster, "Control out"=w536:refnum<class "Control.lvclass">)  [unwired: 6 out]
            n309 = Bundle By Name(cluster=w538, "Control"=w536) -> (w537:T20)
            n310 = call <vilib>:"Add State(s) to Queue__jki_lib_state_machine.vi"("State(s) in Front (\"\")"="Preview", "State(s) in (\"\")"=w541) -> ("States Out"=w540:string)  [unwired: 1 in, 12 out]
          }
          event User Event {
            n311 = event-data() -> ("Style"=w542:u16)  [unwired: 5 out]
            n312 = Unbundle By Name(w548) -> ("Control"=w544:refnum<class "Control.lvclass">)
            n313 = call-dynamic "Write Style.vi"("error in (no error)"=w543, "Style index (-1)"=w542, "Control in"=w544) -> ("error out"=w545:errorcluster, "Control out"=w546:refnum<class "Control.lvclass">)  [unwired: 1 in, 6 out]
            n314 = property on="Button Style" class="Ring (strict)"("Value"=w542) -> ()  [unwired: 2 in, 2 out]
            n315 = Bundle By Name(cluster=w548, "Control"=w546) -> (w547:T20)
            n316 = call <vilib>:"Add State(s) to Queue__jki_lib_state_machine.vi"("State(s) in Front (\"\")"="Preview", "State(s) in (\"\")"=w551) -> ("States Out"=w550:string)  [unwired: 1 in, 12 out]
          }
          event User Event {
            n317 = event-data() -> ("Text Color"=w552:u32)  [unwired: 5 out]
            n318 = Unbundle By Name(w558) -> ("Control"=w554:refnum<class "Control.lvclass">)
            n319 = property on="Text Color" class="ColBox"("Value"=w552) -> ()  [unwired: 2 in, 2 out]
            n320 = call-dynamic "Write Text Color.vi"("error in (no error)"=w553, "Text Color"=w552, "Control.lvclass in"=w554) -> ("error out"=w555:errorcluster, "Control.lvclass out"=w556:refnum<class "Control.lvclass">)  [unwired: 7 out]
            n321 = Bundle By Name(cluster=w558, "Control"=w556) -> (w557:T20)
            n322 = call <vilib>:"Add State(s) to Queue__jki_lib_state_machine.vi"("State(s) in Front (\"\")"="Preview", "State(s) in (\"\")"=w561) -> ("States Out"=w560:string)  [unwired: 1 in, 12 out]
          }
          event User Event {
            # "If the Control Text terminal is not empty, then do not override the user's input."
            n323 = event-data() -> ("Icon (*.png)"=w566:path)  [unwired: 5 out]
            n324 = Unbundle By Name(w579) -> ("Control"=w567:refnum<class "Control.lvclass">)
            n325 = call-poly <userlib>:"Strip Path__ogtk.vi"("path"=w566) -> ("name"=w574:string)  [unwired: 1 out]
            n326 = local read "FALSE Text"() -> (w576:string)
            n327 = call-poly <userlib>:"Strip Path Extension__ogtk.vi"("path"=w574) -> ("root"=w573:string)  [unwired: 1 out]
            n328 = call-dynamic "Load Icon.vi"("error in (no error)"=w572, "Icon path False"=w566, "Control in"=w567) -> ("error out"=w571:errorcluster, "Control out"=w568:refnum<class "Control.lvclass">)  [unwired: 1 in, 6 out]
            n329 = call-poly <userlib>:"To Proper Case__ogtk.vi"("string"=w573) -> ("proper case string"=w577:string)  [unwired: 4 out]
            n330 = property on="Icon source" class="Path"("Value"=w566) -> ()  [unwired: 2 in, 2 out]
            n331 = Empty String/Path?(string/path=w576) -> (empty?=w575:bool)
            n332 = local read "Same decal True/False"() -> (w562:bool)
            n333 = Select(t=w577, s=w575, f=w576) -> (s? t:f=w564:string)
            n334 = local read "TRUE Text"() -> (w565:string)
            n335 = local write "FALSE Text"(w564) -> ()
            n336 = Select(t=w564, s=w562, f=w565) -> (s? t:f=w563:string)
            n337 = call-dynamic "Write Control Text.vi"("error in (no error)"=w571, "True Text"=w563, "False Text"=w564, "Control in"=w568) -> ("error out"=w570:errorcluster, "Control out"=w569:refnum<class "Control.lvclass">)  [unwired: 6 out]
            n338 = Bundle By Name(cluster=w579, "Control"=w569) -> (w578:T20)
            n339 = call <vilib>:"Add State(s) to Queue__jki_lib_state_machine.vi"("State(s) in Front (\"\")"="Preview", "State(s) in (\"\")"=w582) -> ("States Out"=w581:string)  [unwired: 1 in, 12 out]
          }
          event "Zoom Min": Value Change {
            # "Zoomig is set from 0.5 to 2."
            n340 = event-data() -> ()  [unwired: 7 out]
            n341 = Unbundle By Name(w589) -> ("Control"=w586:refnum<class "Control.lvclass">, "user events.Scale Icon"=w585:refnum<user-event>)
            n342 = Generate User Event(user event=w585, event data cluster=0.5 ("event data"), error in=w584) -> (error out=w583:errorcluster)  [unwired: 1 in, 1 out]
            n343 = Bundle By Name(cluster=w589, "Control"=w586) -> (w588:T20)
            n344 = call <vilib>:"Add State(s) to Queue__jki_lib_state_machine.vi"("State(s) in Front (\"\")"="Preview", "State(s) in (\"\")"=w592) -> ("States Out"=w591:string)  [unwired: 1 in, 12 out]
          }
          event "Zoom Max": Value Change {
            # "Zoomig is set from 0.5 to 2."
            n345 = event-data() -> ()  [unwired: 7 out]
            n346 = Unbundle By Name(w599) -> ("Control"=w596:refnum<class "Control.lvclass">, "user events.Scale Icon"=w595:refnum<user-event>)
            n347 = Generate User Event(user event=w595, event data cluster=2.0 ("event data"), error in=w594) -> (error out=w593:errorcluster)  [unwired: 1 in, 1 out]
            n348 = Bundle By Name(cluster=w599, "Control"=w596) -> (w598:T20)
            n349 = call <vilib>:"Add State(s) to Queue__jki_lib_state_machine.vi"("State(s) in Front (\"\")"="Preview", "State(s) in (\"\")"=w602) -> ("States Out"=w601:string)  [unwired: 1 in, 12 out]
          }
          event Panel Close? {
            # "Discard the event because we'll close the front panel ourselves in Macro: Exit"
            # "Close Panel button (pressed) Event\n(this executes Macro: Exit to terminate the VI)"
            n350 = event-data() -> ()  [unwired: 2 out]
            n351 = event-data("Discard?"=TRUE) -> ()  [unwired: 1 in, 1 out]
            n352 = call <vilib>:"Add State(s) to Queue__jki_lib_state_machine.vi"("State(s) in Front (\"\")"="Macro: Exit", "State(s) in (\"\")"=w604) -> ("States Out"=w603:string)  [unwired: 1 in, 12 out]
          }
        }
      }
      frame "---------- Core ----------" {
        # "Do not put any code in this frame.\n(it is a separator no-op)"
        n353 = call <vilib>:"Add State(s) to Queue__jki_lib_state_machine.vi"("State(s) in (\"\")"=w612) -> ("States Out"=w611:string)  [unwired: 2 in, 12 out]
      }
      frame Default {
        w622 = 42 items=["No error", "Argument error", "Memory is full", "Out of zone", "End of file", "File already open", "Generic file I/O error", "File not found", "File permission error", "Disk is full", "Duplicate path", "Too many files open", "System feature not enabled", "Resource file not found", "Cannot add resource", "Resource not found", "Image not found", "Image memory error", "Pen does not exist", "Config type invalid", "Config token not found", "Config parse error", "Config memory error", "Bad external code format", "Bad external code offset", "External code not present", "Null window", "Destroy window error", "Null menu", "Print aborted", "Bad print record", "Print driver error", "Windows error during printing", "Memory error during printing", "Print dialog error", "Generic print error", "Invalid device refnum", "Device not found", "Device parameter error", "Device unit error", "Cannot open device", "Device call aborted", "Generic error", "Cancelled by user", "Object ID too low", "Object ID too high", "Object not in heap", "Unknown heap", "Unknown object (invalid DefProc)", "Unknown object (DefProc not in table)", "Message out of range", "Invalid (null) method", "Unknown message", "Manager call not supported", "Bad address", "Network operation in progress", "Network operation timed out", "Connection is busy", "Network attribute not supported", "Network error", "Address in use", "System out of memory", "Connection aborted", "Connection refused", "Not connected", "Already connected", "Connection closed", "Initialization error (interapplication manager)", "Bad occurrence", "Wait on unbound occurrence handler", "Occurrence queue overflow", "Datalog type conflict", "Unused", "Unrecognized type (interapplication manager)", "Memory corrupt", "Failed to make temporary DLL", "Old CIN version", "Drag socket not found", "Failed to load drop-object", "Failed to register OLE object", "Failed to release OLE object", "Format specifier type mismatch", "Unknown format specifier", "Too few format specifiers", "Too many format specifiers", "Scan failed", "Newer CIN version", "Error converting to variant", "Runtime menu error", "Password tampered", "Variant attribute not found", "Incompatible variant data type", "Event data is not available", "Event Store is not present", "Occurrence is not found", "Event Queue is not created", "Event info is not available", "Refnum passed is NULL", "Error retrieving Class GUID", "Error retrieving CoClass GUID", "Error retrieving TypeLib GUID.", "Bad built application magic bytes.", "Specific driver is different from the specific driver associated with the Logical Name.", "There is no session opened to the class driver.", "Max Error", "MAX - Error with config objects", "MAX - Error loading configuration", "MAX - Group not supported"]
        # "Current State"
        # "Do not delete, rename, or modify this frame.\n(this is used to capture unhandled states and typos)"
        # "Handle mistyped state name (developer tool)"
        n354 = Format Into String(format string="Software Exception: Unhandled State \"%s\"." ("message"), error in=w618, w613) -> (resulting string=w621:string, error out=w620:errorcluster)  [unwired: 1 in]
        n355 = call <vilib>:"Error Cluster From Error Code.vi"("show call chain? (False)"=TRUE, "error in (no error)"=w620, "error message (\"\")"=w621, "error code (0)"=w622) -> ("error out"=w619:errorcluster)  [unwired: 5 out]
        n356 = call <vilib>:"Add State(s) to Queue__jki_lib_state_machine.vi"("State(s) in (\"\")"=w617) -> ("States Out"=w616:string)  [unwired: 2 in, 12 out]
      }
      frame "About" {
        n357 = call "About control creator.vi"() -> ()  [unwired: 12 out]
        n358 = call <vilib>:"Add State(s) to Queue__jki_lib_state_machine.vi"("State(s) in (\"\")"=w627) -> ("States Out"=w626:string)  [unwired: 2 in, 12 out]
      }
      frame "Initialize Core Data" {
        # "If panel starts closed or is an EXE or is launched from Tools menu, then close it when we exit"
        # "Do not delete, rename, or modify this frame.\n(this is used to determine panel behavior on exit)"
        # "originally closed?"
        # "exe?"
        n359 = property class="Application" props=["App.MenuLaunchApp", "App.Name"]() -> (error out=w634:errorcluster, "App.MenuLaunchApp"=w632:refnum<vi>)  [unwired: 2 in, 2 out]
        n360 = property class="VI"() -> ("Front Panel.Open"=w641:bool)  [unwired: 2 in, 2 out]
        n361 = property class="App"() -> (reference out=w630:refnum<vi>, "App.Kind"=w640:T12)  [unwired: 2 in, 1 out]
        n362 = control-ref of="Current VI Reference"() -> (w635:refnum<vi>)
        n363 = Not(x=w641) -> (.not. x?=w638:bool)
        n364 = Equal?(x=w640, y=T12."Run Time System" ("Application:Kind")) -> (x = y?=w637:bool)
        n365 = Unbundle By Name(w634) -> ("status"=w633:bool)
        n366 = Not(x=w633) -> (.not. x?=w631:bool)
        n367 = Or(x=w638, y=w637) -> (x .or. y?=w629:bool)
        n368 = Or(x=w629, y=w631) -> (x .or. y?=w628:bool)
        n369 = Bundle By Name(cluster=w636, "Core.Current VI Reference"=w635, "Core.Close Panel on Exit?"=w628, "Core.NI.LV.Dialog namespace"=w631, "Core.Menu Launch:App"=w632, "Core.Local App"=w630) -> (w643:T20)
        n370 = call <vilib>:"Add State(s) to Queue__jki_lib_state_machine.vi"("State(s) in (\"\")"=w645) -> ("States Out"=w644:string)  [unwired: 2 in, 12 out]
      }
      frame "Error Handler" {
        # "Handle any errors here.\nYou can also output any states to clean-up after errors occur"
        # "Clear error"
        n371 = Unbundle By Name(w647) -> ("code"=w650:i32)
        n372 = Unbundle By Name(w652) -> ("Errors"=w651:T21)
        n373 = for {
          tunnel: w651 -> [w668] mode=indexing
          tunnel: w650 -> [w669]
          tunnel: [w668] -> w648
          tunnel: [w667] -> w649
          stop <- w667 stop-if-true
          n374 = Unbundle By Name(w668) -> ("code"=w670:i32)
          n375 = Equal?(x=w670, y=w669) -> (x = y?=w667:bool)
        }
        n376 = case shown="True" w649 {
          tunnel: w648 -> [_ w666]
          tunnel: w647 -> [w657 _]
          tunnel: ["/* Post Error States" w662] -> w646
          frame False {
            # "Unhandled Error -- Display it"
            n377 = call <vilib>:"General Error Handler.vi"("error in (no error)"=w657) -> ()  [unwired: 1 in, 14 out]
          }
          frame True {
            # "Existing error code: look in the file for description\nand display it.\n\nIf error is critical, exit safely. Otherwise clear error and continue."
            n378 = Unbundle By Name(w666) -> ("Critical"=w665:bool, "Long"=w660:string, "code"=w661:i32)  [unwired: 1 out]
            n379 = Format Into String(format string="Error %d.\n\n%s", w661, w660) -> (resulting string=w659:string)  [unwired: 2 in, 1 out]
            n380 = One Button Dialog(message=w659) -> ()  [unwired: 2 out]
            n381 = Select(t="Macro: Exit", s=w665, f="/* Post Error States") -> (s? t:f=w662:string)
          }
        }
        n382 = call <vilib>:"Add State(s) to Queue__jki_lib_state_machine.vi"("State(s) in Front (\"\")"=w646, "State(s) in (\"\")"=w655) -> ("States Out"=w654:string)  [unwired: 1 in, 12 out]
      }
      frame "Error" {
        # "Add an error code to the queue.\n(Will be processed by Error Handler case)"
        n383 = Decimal String To Number(string=w678, default (0L)=0 ("default (0 I32)")) -> (number=w672:i32)  [unwired: 2 out]
        n384 = Unbundle By Name(w677) -> ("Errors"=w673:T21)
        n385 = for {
          tunnel: w673 -> [w685] mode=indexing
          tunnel: w672 -> [w682]
          tunnel: [w681] -> w671
          stop <- w683 stop-if-true
          n386 = Unbundle By Name(w685) -> ("Short"=w681:string, "code"=w684:i32)
          n387 = Equal?(x=w684, y=w682) -> (x = y?=w683:bool)
        }
        n388 = Bundle By Name(cluster=errorcluster {"status"=TRUE, "code"=0, "source"=""} ("error out"), "source"=w671, "code"=w672) -> (w674:errorcluster)
        n389 = call <vilib>:"Add State(s) to Queue__jki_lib_state_machine.vi"("State(s) in (\"\")"=w680) -> ("States Out"=w679:string)  [unwired: 2 in, 12 out]
      }
      frame "Exit" {
        # "Do not put any code in this frame.\n(No errors that occur here will be handled.)"
        n390 = Generate User Event(user event=w687, event data cluster=TRUE ("event data")) -> ()  [unwired: 2 in, 2 out]
        n391 = call <vilib>:"Add State(s) to Queue__jki_lib_state_machine.vi"("State(s) in (\"\")"=w692) -> ("States Out"=w691:string)  [unwired: 2 in, 12 out]
      }
      frame "---------- Data ----------" {
        # "Do not put any code in this frame.\n(It is a separator no-op. You can make a copy of this frame to create a new Data frame)"
        n392 = call <vilib>:"Add State(s) to Queue__jki_lib_state_machine.vi"("State(s) in (\"\")"=w696) -> ("States Out"=w695:string)  [unwired: 2 in, 12 out]
      }
      frame "Data: Initialize" {
        w697 = T4 {"Horizontal"=0, "Vertical"=0}  # drop pos
        w699 = cluster{"fade":i32, "droplabel":bool} {"fade"=750, "droplabel"=FALSE}  # config
        w700 = T22 {"Action"=4, "Orientations"=14, "Icon (*.png)"=path "", "Control Text"="", "Style"=0, "Text Color"=0, "Scale"=1.0, "Close afterwards"=FALSE}  # last state
        w698 = path ""  # file in tmp dir
        w702 = T21 []  # Errors
        w703 = refnum<class "Control.lvclass"> refnum  # Control
        w704 = T23 {"Current VI Reference"=refnum, "Close Panel on Exit?"=FALSE, "NI.LV.Dialog namespace"=FALSE, "Menu Launch:App"=refnum, "Local App"=refnum}  # Core
        # "Initialize the shift-register data, here.\n(data names are defined by what you wire into the bundle function)"
        n393 = Bundle("Core"=w704, "Control"=w703, "Errors"=w702, "user events"=w701, "last state"=w700, "config"=w699, "file in tmp dir"=w698, "drop pos"=w697) -> (w706:T20)  [unwired: 1 out]
        n394 = call <vilib>:"Add State(s) to Queue__jki_lib_state_machine.vi"("State(s) in (\"\")"=w708) -> ("States Out"=w707:string)  [unwired: 2 in, 12 out]
      }
      frame "Data: Cleanup" {
        # "If not found in config.ini file, then set to default value."
        # "Cleanup any data and references, here.\n(this is called automatically, by the Macro: Exit)"
        n395 = Unbundle By Name(w728) -> ("Core.Current VI Reference"=w730:refnum<vi>)
        n396 = Unbundle(w711) -> ("Event Registration Refnum"=w710:refnum<event-registration>, "Event Registration Refnum"=w709:refnum<event-registration>)
        n397 = Unregister For Events(event registration refnum=w709) -> ()  [unwired: 1 in, 1 out]
        n398 = Unregister For Events(event registration refnum=w710) -> ()  [unwired: 1 in, 1 out]
        n399 = Close Reference(reference=w730, error in (no error)=w729) -> (error out=w719:errorcluster)
        n400 = call <userlib>:"Current VI's Path__ogtk.vi"() -> ("Current VI's Path (+ Relative)"=w724:path)  [unwired: 1 out]
        n401 = call <userlib>:"Current VIs Parent Directory__ogtk.vi"("Relative path (.)"=path "config.ini") -> ("Parent Directory (+ Relative)"=w725:path)  [unwired: 4 out]
        n402 = call-poly <userlib>:"Strip Path__ogtk.vi"("path"=w724) -> ("name"=w713:string)  [unwired: 1 out]
        n403 = call <vilib>:"Open Config Data (compatibility).vi"("error in (no error)"=w719, "configuration file path"=w725) -> ("error out"=w722:errorcluster, "refnum"=w723:T24)  [unwired: 7 in, 1 out]
        n404 = call-poly <vilib>:"Read Key.vi"("section"=w713, "error in (no error)"=w722, "default value"="750", "key"="fade", "refnum"=w723) -> ("error out"=w714:errorcluster, "found?"=w712:bool, "refnum out"=w715:T24)  [unwired: 1 in, 3 out]
        n405 = case shown="False" w712 {
          tunnel: [w739 w741] -> w717
          tunnel: [w738 w740] -> w716
          tunnel: w715 -> [w737 w741]
          tunnel: w714 -> [w736 w740]
          tunnel: w713 -> [w735 _]
          frame False {
            n406 = call-poly <vilib>:"Write Key.vi"("section"=w735, "error in (no error)"=w736, "value"="750", "key"="fade", "refnum"=w737) -> ("error out"=w738:errorcluster, "refnum out"=w739:T24)  [unwired: 1 in, 4 out]
          }
          frame True {
          }
        }
        n407 = call <vilib>:"Close Config Data.vi"("error in (no error)"=w716, "refnum"=w717) -> ("error out"=w718:errorcluster)  [unwired: 1 in, 8 out]
        n408 = call <vilib>:"Add State(s) to Queue__jki_lib_state_machine.vi"("State(s) in Front (\"\")"="" ("State(s) in Front (\"\")"), "State(s) in (\"\")"=w732) -> ("States Out"=w731:string)  [unwired: 1 in, 12 out]
      }
      frame "---------- UI ----------" {
        # "Do not put any code in this frame.\n(It is a separator no-op. You can make a copy of this frame to create a new UI frame)"
        n409 = call <vilib>:"Add State(s) to Queue__jki_lib_state_machine.vi"("State(s) in (\"\")"=w745) -> ("States Out"=w744:string)  [unwired: 2 in, 12 out]
      }
      frame "UI: Initialize" {
        # "Initialize the VI's behavior"
        # "Initialize the User Interface, here.\n(this is called automatically, by the Macro: Init)"
        n410 = Unbundle By Name(w748) -> ("Core.Current VI Reference"=w754:refnum<vi>)
        n411 = property class="VI"(reference=w754, "Front Panel.ShowMenuBar"=TRUE ("Front Panel Window:Show Menu Bar"), "Front Panel.TitleBarVis"=TRUE ("Front Panel Window:Show Menu Bar"), "Front Panel.Minimizeable"=TRUE ("Front Panel Window:Show Menu Bar"), "Front Panel.Resizeable"=FALSE ("Front Panel Window:Show Menu Bar"), "Front Panel.Closeable"=TRUE ("Front Panel Window:Show Menu Bar")) -> ()  [unwired: 1 in, 2 out]
        n412 = call <vilib>:"Add State(s) to Queue__jki_lib_state_machine.vi"("State(s) in Front (\"\")"="UI: Read Config\nUI: Transparency >> TRUE\nUI: FadeIn\nControl: Read error list\nUI: List Projects\nUI: List Open FPs" ("State(s) in Front (\"\")"), "State(s) in (\"\")"=w756) -> ("States Out"=w755:string)  [unwired: 1 in, 12 out]
      }
      frame "UI: Read Config" {
        n413 = Unbundle By Name(w759) -> ("config"=w760:cluster{"fade":i32, "droplabel":bool})
        n414 = call <userlib>:"Current VIs Parent Directory__ogtk.vi"("Relative path (.)"=path "config.ini") -> ("Parent Directory (+ Relative)"=w764:path)  [unwired: 4 out]
        n415 = call <userlib>:"Current VI's Path__ogtk.vi"() -> ("Current VI's Path (+ Relative)"=w763:path)  [unwired: 1 out]
        n416 = call-poly <userlib>:"Strip Path__ogtk.vi"("path"=w763) -> ("name"=w766:string)  [unwired: 1 out]
        n417 = call <vilib>:"Open Config Data (compatibility).vi"("error in (no error)"=w762, "configuration file path"=w764) -> ("error out"=w772:errorcluster, "refnum"=w767:T24)  [unwired: 7 in, 1 out]
        n418 = call <userlib>:"Set Data Name__ogtk.vi"("error in (no error)"=w772, "Data Name"=w766, "Data"=w760) -> ("error out"=w771:errorcluster, "Renamed Data"=w768:variant)  [unwired: 7 out]
        n419 = call <userlib>:"Read INI Cluster__ogtk.vi"("error in (no error)"=w771, "INI Fomatted Cluster Type"=w768, "refnum"=w767) -> ("error out"=w770:errorcluster, "INI Fomatted Cluster"=w773:variant, "dup refnum"=w769:T24)  [unwired: 6 out]
        n420 = Variant To Data(type=w760, Variant=w773) -> (data=w757:cluster{"fade":i32, "droplabel":bool})  [unwired: 1 in, 1 out]
        n421 = call <vilib>:"Close Config Data.vi"("error in (no error)"=w770, "refnum"=w769) -> ("error out"=w761:errorcluster)  [unwired: 1 in, 8 out]
        n422 = Bundle By Name(cluster=w759, "config"=w757) -> (w758:T20)
        n423 = call <vilib>:"Add State(s) to Queue__jki_lib_state_machine.vi"("State(s) in (\"\")"=w775) -> ("States Out"=w774:string)  [unwired: 2 in, 12 out]
      }
      frame "UI: Transparency" {
        # "if error ==> opaque"
        # "Initialize the User Interface, here.\n(this is called automatically, by the Macro: Init)"
        n424 = Unbundle By Name(w787) -> ("Core.Current VI Reference"=w786:refnum<vi>)
        n425 = Scan From String(format string="%s", input string=w785, default 1=FALSE) -> (error out=w779:errorcluster, output 1=w782:bool)  [unwired: 2 in, 2 out]
        n426 = Select(t=u8 0, s=w779, f=u8 100) -> (s? t:f=w776:u8)
        n427 = call-poly "SetTransparency(Polymorphic).vi"("error in"=w781, "Run VI Transparently (T)"=w782, "Transparency (%)"=w776, "VI Reference (calling VI)"=w786) -> ("error out"=w780:errorcluster)  [unwired: 7 out]
        n428 = call <vilib>:"Add State(s) to Queue__jki_lib_state_machine.vi"("State(s) in (\"\")"=w789) -> ("States Out"=w788:string)  [unwired: 2 in, 12 out]
      }
      frame "UI: FadeIn" {
        # "Initialize the User Interface, here.\n(this is called automatically, by the Macro: Init)"
        n429 = Unbundle By Name(w794) -> ("Core.Current VI Reference"=w793:refnum<vi>, "config.fade"=w792:i32)
        n430 = call-poly "Fade In(Polymorphic).vi"("error in"=w791, "Fade time (ms)"=w792, "VI Reference (calling VI)"=w793) -> ("error out"=w790:errorcluster)  [unwired: 1 in, 7 out]
        n431 = call <vilib>:"Add State(s) to Queue__jki_lib_state_machine.vi"("State(s) in (\"\")"=w796) -> ("States Out"=w795:string)  [unwired: 2 in, 12 out]
      }
      frame "UI: FadeOut" {
        # "Initialize the User Interface, here.\n(this is called automatically, by the Macro: Init)"
        n432 = Unbundle By Name(w803) -> ("Core.Current VI Reference"=w800:refnum<vi>, "config.fade"=w799:i32)
        n433 = call-poly "Fade Out(Polymorphic).vi"("error in"=w798, "Fade time (ms)"=w799, "VI Reference (calling VI)"=w800) -> ("error out"=w797:errorcluster)  [unwired: 1 in, 7 out]
        n434 = call <vilib>:"Add State(s) to Queue__jki_lib_state_machine.vi"("State(s) in (\"\")"=w802) -> ("States Out"=w801:string)  [unwired: 2 in, 12 out]
      }
      frame "UI: Cursor Set" {
        # "Argument"
        # "Set and Unset Cursor Busy.\n(Usage: \"UI: Cursor Set >> Busy|Idle\")"
        n435 = case shown="\"Idle\", Default" w806 {
          tunnel: w808 -> [w811 w813]
          tunnel: [w810 w812] -> w807
          frame "Idle", Default {
            n436 = call <vilib>:"Unset Busy.vi"("error in (no error)"=w811) -> ("error out"=w810:errorcluster)  [unwired: 1 in, 9 out]
          }
          frame "Busy" {
            n437 = call <vilib>:"Set Busy.vi"("error in (no error)"=w813) -> ("error out"=w812:errorcluster)  [unwired: 3 in, 7 out]
          }
        }
        n438 = call <vilib>:"Add State(s) to Queue__jki_lib_state_machine.vi"("State(s) in (\"\")"=w805) -> ("States Out"=w804:string)  [unwired: 2 in, 12 out]
      }
      frame "UI: Front Panel State" {
        # "Argument"
        # "Set Front Panel Open or Closed\n(Usage: \"UI: Front Panel State >> Open|Close\")"
        n439 = Unbundle By Name(w818) -> ("Core.Current VI Reference"=w817:refnum<vi>)
        n440 = case shown="\"Open\", Default" w816 {
          tunnel: w820 -> [w824 w837]
          tunnel: [w826 w838] -> w819
          tunnel: w817 -> [w825 w835]
          frame "Open", Default {
            n441 = property class="VI"(reference=w825, error in=w824) -> (reference out=w822:refnum<vi>, error out=w823:errorcluster, "Front Panel.Open"=w821:bool)
            n442 = case shown="False" w821 {
              tunnel: [w829 w832] -> w826
              tunnel: w823 -> [w828 w832]
              tunnel: w822 -> [w827 _]
              frame False {
                n443 = invoke class="VI" method="FP.Open"(reference=w827, error in=w828, "Activate"=TRUE, "State"=T13."Standard") -> (error out=w829:errorcluster)  [unwired: 1 in, 4 out]
              }
              frame True {
              }
            }
          }
          frame "Close" {
            n444 = property class="VI"(reference=w835, error in=w837) -> (reference out=w834:refnum<vi>, error out=w836:errorcluster, "Front Panel.Open"=w833:bool)
            n445 = case shown="True" w833 {
              tunnel: [w839 w842] -> w838
              tunnel: w836 -> [w839 w841]
              tunnel: w834 -> [_ w840]
              frame False {
              }
              frame True {
                n446 = invoke class="VI" method="FP.Close"(reference=w840, error in=w841) -> (error out=w842:errorcluster)  [unwired: 1 in, 2 out]
              }
            }
          }
        }
        n447 = call <vilib>:"Add State(s) to Queue__jki_lib_state_machine.vi"("State(s) in (\"\")"=w814) -> ("States Out"=w815:string)  [unwired: 2 in, 12 out]
      }
      frame "UI: List Projects" {
        # "List all projects currently in memory in the same application instance as the caller of this utility."
        n448 = Unbundle By Name(w845) -> ("Core.Menu Launch:App"=w847:refnum<vi>, "Core.NI.LV.Dialog namespace"=w848:bool, "Core.Local App"=w846:refnum<vi>)
        n449 = Select(t=w847, s=w848, f=w846) -> (s? t:f=w844:refnum<vi>)
        n450 = property class="App"(reference=w844) -> ("Project"=w850:refnum<vi>[])  [unwired: 1 in, 2 out]
        n451 = for {
          tunnel: [w862] -> w851 mode=indexing
          tunnel: w850 -> [w861] mode=indexing
          tunnel: [w860] -> w849 mode=indexing
          n452 = property class="Project"(reference=w861) -> (reference out=w860:refnum<vi>, "Name"=w862:string)  [unwired: 1 in, 1 out]
        }
        n453 = Array Size(array=w850) -> (size(s)=w853:i32)
        n454 = Greater Than 0?(x=w853) -> (x > 0?=w843:bool)
        n455 = Close Reference(reference=w849) -> ()  [unwired: 1 in, 1 out]
        n456 = Select(t=u8 0 ("Disabled"), s=w843, f=u8 2 ("Disabled")) -> (s? t:f=w856:u8)
        n457 = property on="Projects" class="Ring (strict)"("Strings []"=w851, "Value"=0, "Disabled"=w856) -> ()  [unwired: 2 in, 2 out]
        n458 = property on="Add to Project" class="Bool (strict)"("Disabled"=w856) -> ()  [unwired: 2 in, 2 out]
        n459 = call <vilib>:"Add State(s) to Queue__jki_lib_state_machine.vi"("State(s) in (\"\")"=w859) -> ("States Out"=w858:string)  [unwired: 2 in, 12 out]
      }
      frame "UI: List Open FPs" {
        w877 = u16 0 items=[""] ("Front Panels")
        # "Disable \"Drop on FP\" option\nif no idle FPs are opened."
        # "keep only Idle front panels to remove this VI,  \"probe VIs\" and\nVIs that are not in a state for scripting to work."
        # "ADAPTED FROM: \nList Open Front Panels.vi\nTO LIST ALL OPEN FRONT PANELS IN THE SELECTED APPLICATION INSTANCE\n\nReturns an array of the names of all VIs in memory whose front panels are open.\n\nPlease visit http://www.OpenG.org to learn about the\nOpen Source LabVIEW software movement.\n\nNOTICE -- YOU MUST LEAVE THIS NOTICE IN PLACE.  PER THE TERMS OF THE LICENSE BELOW, YOU MAY SUBLICENSE THIS SOFTWARE \nIN ANY WAY THAT DOES NOT CONFLICT WITH THIS LICENSE.\n\n### BSD License (http://www.opensource.org/licenses/bsd-license.php) Begin ###\n \nCopyright (c) 2002, Jim Kring <jim@jimkring.com>\n\nAll rights reserved.\n\nRedistribution and use in source and binary forms, with or without modification, are permitted provided that the following conditions are met:\n\n    * Redistributions of source code must retain the above copyright notice, this list of conditions and the following disclaimer.\n    * Redistributions in binary form must reproduce the above copyright notice, this list of conditions and the following disclaimer in the \n       documentation and/or other materials provided with the distribution.\n    * Neither the name of SciWare, James Kring, Inc., nor the names of its contributors may be used to endorse or promote products derived \n       from this software without specific prior written permission.\n\nTHIS SOFTWARE IS PROVIDED BY THE COPYRIGHT HOLDERS AND CONTRIBUTORS \"AS IS\" AND ANY EXPRESS OR IMPLIED WARRANTIES, \nINCLUDING, BUT NOT LIMITED TO, THE IMPLIED WARRANTIES OF MERCHANTABILITY AND FITNESS FOR A PARTICULAR PURPOSE ARE \nDISCLAIMED. IN NO EVENT SHALL THE COPYRIGHT OWNER OR CONTRIBUTORS BE LIABLE FOR ANY DIRECT, INDIRECT, INCIDENTAL,\n SPECIAL, EXEMPLARY, OR CONSEQUENTIAL DAMAGES (INCLUDING, BUT NOT LIMITED TO, PROCUREMENT OF SUBSTITUTE GOODS OR \nSERVICES; LOSS OF USE, DATA, OR PROFITS; OR BUSINESS INTERRUPTION) HOWEVER CAUSED AND ON ANY THEORY OF LIABILITY, \nWHETHER IN CONTRACT, STRICT LIABILITY, OR TORT (INCLUDING NEGLIGENCE OR OTHERWISE) ARISING IN ANY WAY OUT OF THE USE \nOF THIS SOFTWARE, EVEN IF ADVISED OF THE POSSIBILITY OF SUCH DAMAGE.\n\n### BSD License End ###"
        n460 = Unbundle By Name(w867) -> ("Core.Menu Launch:App"=w865:refnum<vi>, "Core.NI.LV.Dialog namespace"=w866:bool, "Core.Local App"=w864:refnum<vi>)
        n461 = Select(t=w865, s=w866, f=w864) -> (s? t:f=w868:refnum<vi>)
        n462 = property class="App"(reference=w868) -> (reference out=w869:refnum<vi>, "Application:All VIs In Memory"=w871:string[])  [unwired: 1 in, 1 out]
        n463 = for {
          tunnel: w871 -> [w891] mode=indexing
          shift-right: [w889] -> w863
          shift-left: string[] [] ("Application:All VIs In Memory") -> [w890]
          tunnel: w869 -> [w887]
          tunnel: [w881] -> _ mode=indexing
          n464 = Open VI Reference(application reference (local)=w887, vi path=w891, options=2) -> (vi reference=w895:refnum<vi>, error out=w894:errorcluster)  [unwired: 1 in, 2 out]
          n465 = property class="VI"(reference=w895, error in=w894) -> (reference out=w893:refnum<vi>, error out=w892:errorcluster, "Front Panel Window:Open"=w883:bool, "Exec.State"=w886:T14)
          n466 = Equal?(x=w886, y=T14."Idle" ("Execution:State")) -> (x = y?=w884:bool)
          n467 = And(x=w883, y=w884) -> (x .and. y?=w882:bool)
          n468 = case shown="True" w882 {
            tunnel: w891 -> [_ w899]
            tunnel: w890 -> [w896 w898]
            tunnel: [w896 w897] -> w889
            frame False {
            }
            frame True {
              n469 = Build Array (concatenate)(w898, w899) -> (w897:string[])
            }
          }
          n470 = Close Reference(reference=w893, error in (no error)=w892) -> (error out=w881:errorcluster)
        }
        n471 = Array Size(array=w863) -> (size(s)=w872:i32)
        n472 = Greater Than 0?(x=w872) -> (x > 0?=w875:bool)
        n473 = Select(t=u8 0 ("Disabled"), s=w875, f=u8 2 ("Disabled")) -> (s? t:f=w876:u8)
        n474 = property on="Front Panels" class="Ring (strict)"("Value"=w877, "Strings []"=w863, "Disabled"=w876) -> ()  [unwired: 2 in, 2 out]
        n475 = property on="Drop on Front Panel" class="Bool (strict)"("Value"=w875, "Disabled"=w876) -> ()  [unwired: 2 in, 2 out]
        n476 = call <vilib>:"Add State(s) to Queue__jki_lib_state_machine.vi"("State(s) in (\"\")"=w880) -> ("States Out"=w879:string)  [unwired: 2 in, 12 out]
      }
      frame "---------- Macro ----------" {
        # "Do not put any code in this frame.\n(It is a separator no-op. You can make a copy of this frame to create a new Macro frame)"
        n477 = call <vilib>:"Add State(s) to Queue__jki_lib_state_machine.vi"("State(s) in (\"\")"=w903) -> ("States Out"=w902:string)  [unwired: 2 in, 12 out]
      }
      frame "Macro: Initialize" {
        w904 = "Data: Initialize\nInitialize Core Data\nUI: Initialize\nUI: Front Panel State >> Open\nControl: Init"  # Data: Initialize Initialize Core Data UI: Initialize UI: Front Panel State >> Open Control: Init
        # "Initialization Macro\n(This is called once, when the VI starts)"
        n478 = call <vilib>:"Add State(s) to Queue__jki_lib_state_machine.vi"("State(s) in Front (\"\")"=w904, "State(s) in (\"\")"=w908) -> ("States Out"=w907:string)  [unwired: 1 in, 12 out]
      }
      frame "Macro: Exit" {
        # "Exit Macro\n(This is called once, when the VI exits)"
        n479 = Unbundle By Name(w911) -> ("Core.Close Panel on Exit?"=w917:bool)  [unwired: 1 out]
        n480 = Select(t="UI: Front Panel State >> Close", s=w917, f="") -> (s? t:f=w914:string)
        n481 = call <vilib>:"Add State(s) to Queue__jki_lib_state_machine.vi"("State(s) in Front (\"\")"="Control: Save Config\nUI: FadeOut", "State(s) in (\"\")"=w914, "State(s) at Back (\"\")"="Data: Cleanup\nExit") -> ("States Out"=w912:string)  [unwired: 12 out]
        n482 = call <vilib>:"Add State(s) to Queue__jki_lib_state_machine.vi"("State(s) in Front (\"\")"=w912, "State(s) in (\"\")"=w919) -> ("States Out"=w918:string)  [unwired: 1 in, 12 out]
      }
      frame "---------- Control ----------" {
        # "Template Separator\n(You can make a copy of, or modify, this frame)"
        n483 = call <vilib>:"Add State(s) to Queue__jki_lib_state_machine.vi"("State(s) in (\"\")"=w923) -> ("States Out"=w922:string)  [unwired: 2 in, 12 out]
      }
      frame "Center on Pane" {
        n484 = control-ref of="PREVIEW"() -> (w932:refnum<vi>)
        n485 = call "FindOwningPane.vi"("error in (no error)"=w931, "GObject"=w932) -> ("error out"=w936:errorcluster, "Owning Pane"=w937:refnum<vi>, "GObject dup"=w935:refnum<vi>)  [unwired: 7 out]
        n486 = property class="Pane"(reference=w937, error in=w936, "Origin"=T4 {"Horizontal"=0, "Vertical"=0}) -> (reference out=w927:refnum<vi>, error out=w926:errorcluster, "ContentBnds"=w939:T8)
        n487 = Close Reference(reference=w927, error in (no error)=w926) -> (error out=w925:errorcluster)
        n488 = call "Calculate_GObject_Rectangle.vi"("error in"=w925, "GObject ref"=w935) -> ("error out"=w924:errorcluster, "Rectangle"=w933:T9, "GObject ref dup"=w934:refnum<vi>)  [unwired: 7 out]
        n489 = call "Snap to Center.vi"("Fixed Rect"=w939, "Rect"=w933) -> ("TopLeft point"=w938:cluster{"x":i32, "y":i32})  [unwired: 9 out]
        n490 = property class="GObj"(reference=w934, error in=w924, "Position"=w938) -> (reference out=w930:refnum<vi>, error out=w929:errorcluster)
        n491 = Close Reference(reference=w930, error in (no error)=w929) -> (error out=w928:errorcluster)
        n492 = call <vilib>:"Add State(s) to Queue__jki_lib_state_machine.vi"("State(s) in (\"\")"=w943) -> ("States Out"=w942:string)  [unwired: 2 in, 12 out]
      }
      frame "Preview" {
        # "Resize and Display"
        # "Add the other states"
        # "Get first state"
        # "Generate a preview in the right-end side of the interface, centered on Pane.\nIf many button states are found, then they will be concatenated to a single picture."
        n493 = Unbundle By Name(w952) -> ("Control"=w953:refnum<class "Control.lvclass">)
        n494 = call-dynamic "Preview Control States.vi"("error in"=w947, "Control in"=w953) -> ("error out"=w946:errorcluster, "States preview"=w954:picture[], "Control out"=w950:refnum<class "Control.lvclass">)  [unwired: 7 out]
        n495 = Delete From Array(array=w954, length=1, index=0) -> (deleted portion=w959:picture[], array with subset deleted=w960:picture[])
        n496 = Index Array(array=w959) -> (element=w956:picture)  [unwired: 1 in]
        n497 = call <vilib>:"Picture to Pixmap.vi"("Background Color"=u32 16448250 ("Color Box"), "depth"=24, "picture"=w956) -> ("image data"=w964:T19)  [unwired: 1 in, 7 out]
        n498 = for {
          tunnel: w960 -> [w975] mode=indexing
          shift-right: [w971] -> w961
          shift-left: w964 -> [w970]
          n499 = call <vilib>:"Picture to Pixmap.vi"("Background Color"=u32 16448250 ("Color Box"), "picture"=w975) -> ("image data"=w969:T19)  [unwired: 2 in, 7 out]
          n500 = call <vilib>:"Unflatten Pixmap.vi"("image data"=w970) -> ("24-bit pixmap"=w974:u32[][])  [unwired: 10 out]
          n501 = call <vilib>:"Unflatten Pixmap.vi"("image data"=w969) -> ("24-bit pixmap"=w973:u32[][])  [unwired: 10 out]
          n502 = Build Array (concatenate)(w974, w973) -> (w972:u32[][])
          n503 = call <vilib>:"Flatten Pixmap.vi"("24-bit pixmap"=w972) -> ("image data"=w971:T19)  [unwired: 5 in, 5 out]
        }
        n504 = control-ref of="PREVIEW"() -> (w949:refnum<vi>)
        n505 = Unbundle By Name(w961) -> ("Rectangle"=w962:T9)
        n506 = call <vilib>:"Draw Flattened Pixmap.vi"("image data"=w961) -> ("new picture"=→"PREVIEW":picture)  [unwired: 1 in, 7 out]
        n507 = call <vilib>:"RectSize.vi"("rect"=w962) -> ("point"=w963:cluster{"x":i16, "y":i16})
        n508 = property class="Pict"(reference=w949, error in=w946, "Draw Area Size"=w963) -> (error out=w944:errorcluster)  [unwired: 1 out]
        n509 = Bundle By Name(cluster=w952, "Control"=w950) -> (w951:T20)
        n510 = call <vilib>:"Add State(s) to Queue__jki_lib_state_machine.vi"("State(s) in Front (\"\")"="Center on Pane", "State(s) in (\"\")"=w967) -> ("States Out"=w966:string)  [unwired: 1 in, 12 out]
      }
      frame "Control: Read error list" {
        # "Read the error list from the file."
        n511 = Unbundle By Name(w981) -> ("Control"=w986:refnum<class "Control.lvclass">, "Errors"=w977:T21)
        n512 = Index Array(array=w977) -> (element=w976:T25)  [unwired: 1 in]
        n513 = call <vilib>:"Get LV Class Path.vi"("object"=w986) -> ("error out"=w990:errorcluster, "class path"=w992:path)  [unwired: 1 in, 8 out]
        n514 = while {
          shift-right: [w1018] -> w993
          shift-left: w992 -> [w1020]
          tunnel: w990 -> [_]
          stop <- w1022 stop-if-true
          # "Extracted from OpenG: \n\"Current VI Parent Dir\""
          n515 = call-poly <userlib>:"Strip Path__ogtk.vi"("path"=w1020) -> ("stripped path"=w1018:path)  [unwired: 1 out]
          n516 = File/Directory Info(path=w1018) -> (directory=w1023:bool)  [unwired: 1 in, 6 out]
          n517 = Not A Number/Path/Refnum?(number/path/refnum=w1020) -> (NaN/Path/Refnum?=w1021:bool)
          n518 = Empty String/Path?(string/path=w1020) -> (empty?=w1019:bool)
          n519 = Compound Arithmetic op=OR(w1023, w1021, w1019) -> (w1022:bool)
        }
        n520 = Build Path(base path=w993, name or relative path="errors.txt") -> (appended path=w989:path)
        n521 = call <vilib>:"Open Config Data (compatibility).vi"("configuration file path"=w989) -> ("error out"=w988:errorcluster, "refnum"=w987:T24)  [unwired: 8 in, 1 out]
        n522 = call <vilib>:"Get Section Names.vi"("error in (no error)"=w988, "refnum"=w987) -> ("error out"=w985:errorcluster, "section names"=w978:string[], "refnum out"=w984:T24)  [unwired: 1 in, 6 out]
        n523 = for {
          shift-right: [w1012] -> w983
          shift-left: w984 -> [w1016]
          shift-right: [w1013] -> w982
          shift-left: w985 -> [w1017]
          tunnel: w978 -> [w1006] mode=indexing
          tunnel: [w1015] -> w979 mode=indexing
          tunnel: w976 -> [w1014]
          n524 = Decimal String To Number(string=w1006) -> (number=w997:i32)  [unwired: 3 out]
          n525 = call-poly <vilib>:"Read Key.vi"("section"=w1006, "error in (no error)"=w1017, "default value"=FALSE, "key"="Critical" ("name or relative path"), "refnum"=w1016) -> ("error out"=w1009:errorcluster, "value"=w998:bool, "refnum out"=w1010:T24)  [unwired: 4 out]
          n526 = call-poly <vilib>:"Read Key.vi"("section"=w1006, "error in (no error)"=w1009, "default value"="", "key"="Long" ("name or relative path"), "refnum"=w1010) -> ("error out"=w1008:errorcluster, "value"=w1000:string, "refnum out"=w1011:T24)  [unwired: 1 in, 3 out]
          n527 = call-poly <vilib>:"Read Key.vi"("section"=w1006, "error in (no error)"=w1008, "default value"="", "key"="Short" ("name or relative path"), "refnum"=w1011) -> ("error out"=w1013:errorcluster, "value"=w1001:string, "refnum out"=w1012:T24)  [unwired: 1 in, 3 out]
          n528 = Bundle(cluster=w1014, "code"=w997, "Short"=w1001, "Long"=w1000, "Critical"=w998) -> (w1015:T25)
        }
        n529 = Bundle By Name(cluster=w981, "Errors"=w979) -> (w980:T20)
        n530 = call <vilib>:"Add State(s) to Queue__jki_lib_state_machine.vi"("State(s) in (\"\")"=w996) -> ("States Out"=w995:string)  [unwired: 2 in, 12 out]
        n531 = call <vilib>:"Close Config Data.vi"("error in (no error)"=w982, "refnum"=w983) -> ()  [unwired: 1 in, 9 out]
      }
      frame "Control: Save Temp Control" {
        # "Create a temporary filename for the control to be saved in."
        n532 = Unbundle By Name(w1033) -> ("Control"=w1031:refnum<class "Control.lvclass">)
        n533 = call-dynamic "Read Target path ctl.vi"("Control in"=w1031) -> ("Target path (.ctl)"=w1030:path, "Control out"=w1027:refnum<class "Control.lvclass">)  [unwired: 1 in, 8 out]
        n534 = call <userlib>:"Temporary Filename__ogtk.vi"("pattern (lvtemp%d.tmp)"="temp_control_%d.ctl" ("pattern (all files)"), "sub directory"=path "control") -> ("file in tmp dir"=w1024:path)  [unwired: 1 in, 4 out]
        n535 = call-dynamic "Create Control (to dir).vi"("Target Folder or .ctl"=w1024, "Control in"=w1027) -> ("Control out"=w1028:refnum<class "Control.lvclass">)  [unwired: 1 in, 8 out]
        n536 = call-dynamic "Write Target path ctl.vi"("Target path (.ctl)"=w1030, "Control in"=w1028) -> ("Control out"=w1029:refnum<class "Control.lvclass">)  [unwired: 1 in, 8 out]
        n537 = Bundle By Name(cluster=w1033, "Control"=w1029, "file in tmp dir"=w1024) -> (w1032:T20)
        n538 = call <vilib>:"Add State(s) to Queue__jki_lib_state_machine.vi"("State(s) in (\"\")"=w1036) -> ("States Out"=w1035:string)  [unwired: 2 in, 12 out]
      }
      frame "Control: Prepare batch" {
        # "TO BE ADDED:\n\nWhen preparing for batch processing, launch a VI\nwith VI Server that will calculate the number of PNGs in the\ndirectory recursively while letting this utility run in parallel.\nOtherwise, if the number of files is huge, it could make the\nutility appear to hang indefinitely.\n\nTake only the first PNG for preview."
        n539 = property on="Icon source" class="Path"() -> ("Value"=w1037:path)  [unwired: 2 in, 2 out]
        n540 = Unbundle By Name(w1041) -> ("Control"=w1039:refnum<class "Control.lvclass">)
        n541 = disable-structure shown="Disabled" {
          disable-tunnel: w1037 -> [w1046 _]
          disable-tunnel: "*.png" ("pattern") -> [w1045 _]
          frame Disabled {
            n542 = call <userlib>:"List Directory Recursive__ogtk.vi"("pattern"=w1045, "Path"=w1046) -> ()  [unwired: 3 in, 7 out]
          }
          frame Enabled {
          }
        }
        n543 = Bundle By Name(cluster=w1041, "Control"=w1039) -> (w1040:T20)
        n544 = call <vilib>:"Add State(s) to Queue__jki_lib_state_machine.vi"("State(s) in (\"\")"=w1044) -> ("States Out"=w1043:string)  [unwired: 2 in, 12 out]
      }
      frame "Control: Save Control to Disk" {
        n545 = Unbundle By Name(w1065) -> ("Control"=w1054:refnum<class "Control.lvclass">)
        n546 = property on="Add to Project" class="Bool (strict)"() -> ("Value"=w1047:bool)  [unwired: 2 in, 2 out]
        n547 = case shown="True" w1047 {
          tunnel: [w1077 w1083] -> w1055
          frame False {
            n548 = Call Chain() -> (call chain=w1082:string[])
            n549 = Reverse 1D Array(array=w1082) -> (reversed array=w1081:string[])
            n550 = Index Array(array=w1081) -> (element=w1080:string)  [unwired: 1 in]
            n551 = Open VI Reference(vi path=w1080) -> (vi reference=w1079:refnum<vi>)  [unwired: 1 in, 5 out]
            n552 = property class="VI"(reference=w1079) -> ("Path"=w1078:path)  [unwired: 1 in, 2 out]
            n553 = Strip Path(path=w1078) -> (stripped path=w1077:path)  [unwired: 1 out]
          }
          frame True {
            # "If \"Add to Project\" selected, then set start path to be the \nsame as the project's directory."
            n554 = property on="Projects" class="Ring (strict)"() -> ("Strings []"=w1085:string[], "Value"=w1084:u16)  [unwired: 2 in, 2 out]
            n555 = Index Array(array=w1085, index=w1084) -> (element=w1086:string)
            n556 = call "Get project path.vi"("Project Name"=w1086) -> ("Project path"=w1083:path)
          }
        }
        n557 = local read "FALSE Text"() -> (w1059:string)
        n558 = property on="Button Style" class="Ring (strict)"() -> ("Strings []"=w1063:string[], "Value"=w1062:u16)  [unwired: 2 in, 2 out]
        n559 = Index Array(array=w1063, index=w1062) -> (element=w1061:string)
        n560 = Concatenate Strings(w1061, "_" ("string"), w1059, ".ctl" ("pattern (all files)")) -> (w1056:string)
        n561 = call "File Dialog4"("start path"=w1055, "default name"=w1056, "error in"=w1048, "pattern (all files)"="*.ctl") -> ("selected path"=w1052:path, "cancelled"=w1051:bool, "error out"=w1050:errorcluster)  [unwired: 3 in, 6 out]
        n562 = case shown="False" w1051 {
          tunnel: w1054 -> [w1072 w1076]
          tunnel: [w1074 w1076] -> w1053
          tunnel: w1052 -> [w1070 _]
          tunnel: w1050 -> [w1069 w1075]
          tunnel: [w1073 w1075] -> w1049
          frame False {
            n563 = call-dynamic "Write Target path ctl.vi"("error in (no error)"=w1069, "Target path (.ctl)"=w1070, "Control in"=w1072) -> ("error out"=w1068:errorcluster, "Control out"=w1071:refnum<class "Control.lvclass">)  [unwired: 7 out]
            n564 = call-dynamic "Create Control (to dir).vi"("error in (no error)"=w1068, "Target Folder or .ctl"=w1070, "Control in"=w1071) -> ("error out"=w1073:errorcluster, "Control out"=w1074:refnum<class "Control.lvclass">)  [unwired: 7 out]
          }
          frame True {
          }
        }
        n565 = Bundle By Name(cluster=w1065, "Control"=w1053) -> (w1064:T20)
        n566 = call <vilib>:"Add State(s) to Queue__jki_lib_state_machine.vi"("State(s) in (\"\")"=w1067) -> ("States Out"=w1066:string)  [unwired: 2 in, 12 out]
      }
      frame "Control: Add to FP" {
        w1113 = refnum<vi> refnum  # Boolean
        n567 = Unbundle By Name(w1099) -> ("Control"=w1108:refnum<class "Control.lvclass">, "Core.Menu Launch:App"=w1096:refnum<vi>, "Core.NI.LV.Dialog namespace"=w1097:bool, "Core.Local App"=w1091:refnum<vi>)
        n568 = property on="Front Panels" class="Ring (strict)"(error in=w1106) -> (error out=w1094:errorcluster, "Strings []"=w1110:string[])  [unwired: 1 in, 1 out]
        n569 = Index Array(array=w1110, index="Front Panels") -> (element=w1104:string)
        n570 = Select(t=w1096, s=w1097, f=w1091) -> (s? t:f=w1095:refnum<vi>)
        n571 = Unbundle By Name(w1099) -> ("file in tmp dir"=w1098:path, "config.droplabel"=w1092:bool, "drop pos"=w1089:T4)
        n572 = Open VI Reference(application reference (local)=w1095, vi path=w1104, error in (no error)=w1094) -> (vi reference=w1105:refnum<vi>, error out=w1114:errorcluster)  [unwired: 3 out]
        n573 = property class="VI"(reference=w1105, error in=w1114) -> (reference out=w1111:refnum<vi>, error out=w1112:errorcluster, "Panel"=w1090:refnum<vi>)
        n574 = New VI Object(vi object class=w1113, owner refnum=w1090, position/next to=w1089, 6:w1098, 8:w1112) -> (object refnum=w1103:refnum<vi>, 0:w1102:errorcluster)  [unwired: 3 out]
        n575 = Add(x=T4 {"Horizontal"=20, "Vertical"=20}, y=w1089) -> (x+y=w1087:T4)
        n576 = property class="Bool"(reference=w1103, error in=w1102, "Label.Visible"=w1092) -> (reference out=w1101:refnum<vi>, error out=w1100:errorcluster)
        n577 = Close Reference(reference=w1101, error in (no error)=w1100) -> (error out=w1093:errorcluster)
        n578 = Bundle By Name(cluster=w1099, "Control"=w1108, "drop pos"=w1087) -> (w1115:T20)
        n579 = Close Reference(reference=w1111, error in (no error)=w1093) -> (error out=w1107:errorcluster)
        n580 = call <vilib>:"Add State(s) to Queue__jki_lib_state_machine.vi"("State(s) in (\"\")"=w1117) -> ("States Out"=w1116:string)  [unwired: 2 in, 12 out]
      }
      frame "Control: Add to palette" {
        w1128 = T26 -2 items=["Functions"=-1, "Controls"=-2] ("palette type")
        # "- Add the control to the palette selected. (Defaults to <user.lib>\\_LAVAcr\\CustomControls)"
        # "- Add to dir.mnu file located in <user.lib>\\_LAVAcr\\CustomControls"
        # "TO BE ADDED: \nSet the name to something meaningful (and unique)"
        n581 = Unbundle By Name(w1147) -> ("Control"=w1145:refnum<class "Control.lvclass">, "Core.Menu Launch:App"=w1131:refnum<vi>, "Core.NI.LV.Dialog namespace"=w1132:bool, "Core.Local App"=w1130:refnum<vi>, "file in tmp dir"=w1136:path)
        n582 = call-poly <userlib>:"Strip Path__ogtk.vi"("path"=w1136) -> ("name"=w1119:string)  [unwired: 1 out]
        n583 = call <userlib>:"User Library__ogtk.vi"("Relative path (.)"="Palette") -> ("User Library (+ Relative)"=w1137:path)
        n584 = Select(t=w1131, s=w1132, f=w1130) -> (s? t:f=w1129:refnum<vi>)
        n585 = call <userlib>:"Create Dir if Non-Existant__ogtk.vi"("error in (no error)"=w1140, "Directory Path"=w1137) -> ("error out"=w1141:errorcluster, "dup Directory Path"=w1143:path)  [unwired: 1 in, 7 out]
        n586 = call-poly <userlib>:"Build Path__ogtk.vi"("name or relative path"=w1119, "base path"=w1143) -> ("appended path"=w1144:path)
        n587 = call <userlib>:"User Library__ogtk.vi"("Relative path (.)"=path "_LAVAcr/CustomControls/dir.mnu") -> ("User Library (+ Relative)"=w1135:path)
        n588 = call <userlib>:"Copy with Options__ogtk.vi"("error in (no error)"=w1141, "target path"=w1144, "source path"=w1136) -> ("error out"=w1134:errorcluster, "new path"=w1124:path)  [unwired: 1 in, 6 out]
        n589 = call-poly <userlib>:"Strip Path Extension__ogtk.vi"("path"=w1119) -> ("root"=w1118:string)  [unwired: 1 out]
        n590 = call <vilib>:"Read Palette.vi"("application reference"=w1129, "error in (no error)"=w1134, "palette type"=w1128, "palette path"=w1135) -> ("palette data"=w1125:T27, "duplicate palette path"=w1133:path)  [unwired: 6 out]
        n591 = Unbundle By Name(w1125) -> ("items"=w1121:T29)
        n592 = Bundle By Name(cluster=T15 {"item path"=path "", "library path (.lvlib)"=path "", "use default lvlib palette"=FALSE, "short name"="", "place VI contents"=FALSE, "hide synchronized item"=FALSE, "reserve spot for synch item"=FALSE, "configure when placing VI contents"=FALSE} ("element"), "item path"=w1124, "short name"=w1118) -> (w1122:T15)
        n593 = Build Array (concatenate)(w1121, w1122) -> (w1120:T29)
        n594 = Bundle By Name(cluster=w1125, "items"=w1120) -> (w1126:T27)
        n595 = call <vilib>:"Write Palette.vi"("application reference"=w1129, "palette data"=w1126, "palette type"=w1128, "palette path"=w1133) -> ("error out"=w1127:errorcluster)  [unwired: 1 in, 6 out]
        n596 = Bundle By Name(cluster=w1147, "Control"=w1145) -> (w1146:T20)
        n597 = invoke class="App" method="Refresh Palettes"(error in=w1127) -> (error out=w1139:errorcluster)  [unwired: 2 in, 2 out]
        n598 = call <vilib>:"Add State(s) to Queue__jki_lib_state_machine.vi"("State(s) in (\"\")"=w1149) -> ("States Out"=w1148:string)  [unwired: 2 in, 12 out]
      }
      frame "Control: Add to Project" {
        # "If the file has not been added to disk, then copy the temp control to the\nproject directory with a meaningful name and add it to lvproj file."
        n599 = Unbundle By Name(w1151) -> ("Core.Menu Launch:App"=w1154:refnum<vi>, "Core.NI.LV.Dialog namespace"=w1155:bool, "Core.Local App"=w1153:refnum<vi>, "file in tmp dir"=w1150:path)
        n600 = Unbundle By Name(w1151) -> ("Control"=w1177:refnum<class "Control.lvclass">)
        n601 = local read "FALSE Text"() -> (w1158:string)
        n602 = property on="Button Style" class="Ring (strict)"() -> ("Strings []"=w1162:string[], "Value"=w1161:u16)  [unwired: 2 in, 2 out]
        n603 = call-dynamic "Read Target path ctl.vi"("error in (no error)"=w1169, "Control in"=w1177) -> ("error out"=w1187:errorcluster, "Target path (.ctl)"=w1166:path, "Control out"=w1176:refnum<class "Control.lvclass">)  [unwired: 7 out]
        n604 = Index Array(array=w1162, index=w1161) -> (element=w1160:string)
        n605 = Select(t=w1154, s=w1155, f=w1153) -> (s? t:f=w1152:refnum<vi>)
        n606 = Concatenate Strings(w1160, "_" ("string"), w1158, ".ctl" ("pattern (all files)")) -> (w1156:string)
        n607 = call-poly <userlib>:"File Exists__ogtk.vi"("file path"=w1166) -> ("is directory"=w1171:bool, "exists"=w1172:bool)  [unwired: 6 in]
        n608 = property on="Projects" class="Ring (strict)"() -> ("Strings []"=w1174:string[], "Value"=w1173:u16)  [unwired: 2 in, 2 out]
        n609 = Compound Arithmetic op=AND(invert w1171, w1172) -> (w1167:bool)
        n610 = property class="App"(reference=w1152, error in=w1187) -> ("Project"=w1185:refnum<vi>[])  [unwired: 2 out]
        n611 = Index Array(array=w1174, index=w1173) -> (element=w1175:string)
        n612 = call "Get project path.vi"("Project Name"=w1175) -> ("Project path"=w1170:path)
        n613 = Index Array(array=w1185) -> (element=w1186:refnum<vi>)  [unwired: 1 in]
        n614 = call-poly <userlib>:"Build Path__ogtk.vi"("name or relative path"=w1156, "base path"=w1170) -> ("appended path"=w1188:path)
        n615 = property class="Project"(reference=w1186) -> (reference out=w1183:refnum<vi>, error out=w1179:errorcluster, "My Computer"=w1184:refnum<vi>)  [unwired: 1 in]
        n616 = Close Reference(reference=w1183, error in (no error)=w1179) -> (error out=w1165:errorcluster)
        n617 = case shown="False" w1167 {
          tunnel: w1188 -> [w1196 _]
          tunnel: w1150 -> [w1195 _]
          tunnel: [w1194 w1197] -> w1163
          tunnel: [w1193 w1198] -> w1168
          tunnel: w1166 -> [_ w1198]
          tunnel: w1165 -> [w1192 w1197]
          frame False {
            n618 = call <userlib>:"Copy with Options__ogtk.vi"("error in (no error)"=w1192, "target path"=w1196, "source path"=w1195) -> ("error out"=w1194:errorcluster, "new path"=w1193:path)  [unwired: 1 in, 6 out]
          }
          frame True {
          }
        }
        n619 = invoke class="TargetItem" method="AddFile"(reference=w1184, error in=w1163, "Path"=w1168) -> (reference out=w1182:refnum<vi>, error out=w1180:errorcluster, "AddFile"=w1181:refnum<vi>)  [unwired: 1 in, 1 out]
        n620 = Bundle By Name(cluster=w1151, "Control"=w1176) -> (w1189:T20)
        n621 = Close Reference(reference=w1182, error in (no error)=w1180) -> (error out=w1178:errorcluster)
        n622 = call <vilib>:"Add State(s) to Queue__jki_lib_state_machine.vi"("State(s) in (\"\")"=w1191) -> ("States Out"=w1190:string)  [unwired: 2 in, 12 out]
        n623 = Close Reference(reference=w1181, error in (no error)=w1178) -> (error out=w1164:errorcluster)
      }
      frame "Control: Delete Temp Control" {
        # "Delete the temporary control file."
        n624 = Unbundle By Name(w1208) -> ("Control"=w1206:refnum<class "Control.lvclass">, "file in tmp dir"=w1199:path)
        n625 = call <userlib>:"Delete Recursive__ogtk.vi"("Ignore Read-Only? (FALSE)"=FALSE, "Path"=w1199) -> ("error out"=w1204:errorcluster)  [unwired: 2 in, 7 out]
        n626 = Select(t="Error >> 7002" ("pattern (all files)"), s=w1204, f="") -> (s? t:f=w1201:string)
        n627 = Bundle By Name(cluster=w1208, "Control"=w1206, "file in tmp dir"=path "") -> (w1207:T20)
        n628 = call <vilib>:"Add State(s) to Queue__jki_lib_state_machine.vi"("State(s) in Front (\"\")"=w1201, "State(s) in (\"\")"=w1211) -> ("States Out"=w1210:string)  [unwired: 1 in, 12 out]
      }
      frame "Control: Init" {
        n629 = call "Init_Control.vi"("error in (no error)"=w1219) -> ("error out"=w1223:errorcluster, "App.SaveVersions"=w1220:string[], "Styles strings"=w1216:string[], "Control out"=w1217:refnum<class "Control.lvclass">)  [unwired: 7 out]
        n630 = Empty Array?(array=w1216) -> (empty?=w1215:bool)
        n631 = property on="Button Style" class="Ring (strict)"(error in=w1223, "Strings []"=w1216, "Value"=0) -> (error out=w1221:errorcluster)  [unwired: 1 in, 1 out]
        n632 = Select(t="Error >> 7000", s=w1215, f="Control: Read Config") -> (s? t:f=w1212:string)
        n633 = Bundle By Name(cluster=w1226, "Control"=w1217) -> (w1225:T20)
        n634 = property on="Save for version" class="Ring (strict)"(error in=w1221, "Strings []"=w1220, "Value"=0) -> (error out=w1218:errorcluster)  [unwired: 1 in, 1 out]
        n635 = call <vilib>:"Add State(s) to Queue__jki_lib_state_machine.vi"("State(s) in Front (\"\")"=w1212, "State(s) in (\"\")"=w1228) -> ("States Out"=w1227:string)  [unwired: 1 in, 12 out]
      }
      frame "Control: Read Config" {
        n636 = Unbundle By Name(w1241) -> ("last state"=w1242:T22)
        n637 = call <userlib>:"Current VIs Parent Directory__ogtk.vi"("Relative path (.)"=path "config.ini") -> ("Parent Directory (+ Relative)"=w1256:path)  [unwired: 4 out]
        n638 = call <vilib>:"Open Config Data (compatibility).vi"("error in (no error)"=w1247, "configuration file path"=w1256) -> ("error out"=w1248:errorcluster, "refnum"=w1255:T24)  [unwired: 7 in, 1 out]
        n639 = call <userlib>:"Read INI Cluster__ogtk.vi"("error in (no error)"=w1248, "INI Fomatted Cluster Type"=w1242, "refnum"=w1255) -> ("error out"=w1249:errorcluster, "INI Fomatted Cluster"=w1254:variant, "dup refnum"=w1250:T24)  [unwired: 6 out]
        n640 = Variant To Data(error in=w1249, type=w1242, Variant=w1254) -> (data=w1243:T22, error out=w1235:errorcluster)
        n641 = Bundle By Name(cluster=w1241, "last state"=w1243) -> (w1239:T20)
        n642 = Unbundle By Name(w1239) -> ("Control"=w1238:refnum<class "Control.lvclass">)
        n643 = call-dynamic "Read Text Font.vi"("error in (no error)"=w1235, "Control in"=w1238) -> ("error out"=w1236:errorcluster, "Font"=w1245:T1, "Control out"=w1233:refnum<class "Control.lvclass">)  [unwired: 7 out]
        n644 = call <userlib>:"Read INI Cluster__ogtk.vi"("error in (no error)"=w1236, "INI Fomatted Cluster Type"=w1245, "refnum"=w1250) -> ("error out"=w1253:errorcluster, "INI Fomatted Cluster"=w1251:variant, "dup refnum"=w1252:T24)  [unwired: 6 out]
        n645 = Variant To Data(error in=w1253, type=w1245, Variant=w1251) -> (data=w1231:T1, error out=w1230:errorcluster)
        n646 = call-dynamic "Write Text Font.vi"("error in (no error)"=w1230, "Font"=w1231, "Control in"=w1233) -> ("error out"=w1229:errorcluster, "Control out"=w1232:refnum<class "Control.lvclass">)  [unwired: 7 out]
        n647 = call <vilib>:"Close Config Data.vi"("error in (no error)"=w1229, "refnum"=w1252) -> ("error out"=w1246:errorcluster)  [unwired: 1 in, 8 out]
        n648 = Bundle By Name(cluster=w1239, "Control"=w1232) -> (w1237:T20)
        n649 = call <vilib>:"Add State(s) to Queue__jki_lib_state_machine.vi"("State(s) in Front (\"\")"="Control: Set to Last State", "State(s) in (\"\")"=w1240) -> ("States Out"=w1244:string)  [unwired: 1 in, 12 out]
      }
      frame "Control: Save Config" {
        n650 = Unbundle By Name(w1290) -> ("last state"=w1273:T22, "Control"=w1279:refnum<class "Control.lvclass">)
        n651 = property on="Icon source" class="Path"() -> ("Value"=w1259:path)  [unwired: 2 in, 2 out]
        n652 = call <userlib>:"Current VIs Parent Directory__ogtk.vi"("Relative path (.)"=path "config.ini") -> ("Parent Directory (+ Relative)"=w1296:path)  [unwired: 4 out]
        n653 = call <vilib>:"Open Config Data (compatibility).vi"("error in (no error)"=w1295, "configuration file path"=w1296) -> ("error out"=w1276:errorcluster, "refnum"=w1286:T24)  [unwired: 7 in, 1 out]
        n654 = call-dynamic "Read Action.vi"("error in (no error)"=w1276, "Control in"=w1279) -> ("error out"=w1281:errorcluster, "Action"=w1271:T2, "Control out"=w1280:refnum<class "Control.lvclass">)  [unwired: 7 out]
        n655 = call-dynamic "Read Orientations.vi"("error in (no error)"=w1281, "Control in"=w1280) -> ("error out"=w1284:errorcluster, "Orientations"=w1270:T3, "Control out"=w1283:refnum<class "Control.lvclass">)  [unwired: 7 out]
        n656 = call-dynamic "Read Style.vi"("error in (no error)"=w1284, "Control in"=w1283) -> ("error out"=w1285:errorcluster, "Style index"=w1269:T32, "Control out"=w1282:refnum<class "Control.lvclass">)  [unwired: 7 out]
        n657 = call-dynamic "Read Control Text.vi"("error in (no error)"=w1285, "Control in"=w1282) -> ("error out"=w1261:errorcluster, "Control Text"=w1268:string, "Control out"=w1267:refnum<class "Control.lvclass">)  [unwired: 7 out]
        n658 = call-dynamic "Read Text Color.vi"("error in (no error)"=w1261, "Control.lvclass in"=w1267) -> ("error out"=w1260:errorcluster, "Text Color"=w1263:u32, "Control.lvclass out"=w1266:refnum<class "Control.lvclass">)  [unwired: 7 out]
        n659 = call-dynamic "Read Scale Icon.vi"("error in (no error)"=w1260, "Control in"=w1266) -> ("error out"=w1262:errorcluster, "Scale Icon"=w1264:dbl, "Control out"=w1265:refnum<class "Control.lvclass">)  [unwired: 7 out]
        n660 = Bundle By Name(cluster=w1273, "Scale"=w1264, "Text Color"=w1263, "Control Text"=w1268, "Style"=w1269, "Orientations"=w1270, "Action"=w1271, "Icon (*.png)"=w1259, "Close afterwards"=FALSE) -> (w1272:T22)
        n661 = call <userlib>:"Write INI Cluster__ogtk.vi"("error in (no error)"=w1262, "INI Fomatted Cluster"=w1272, "refnum"=w1286) -> ("error out"=w1275:errorcluster, "dup refnum"=w1289:T24)  [unwired: 1 in, 6 out]
        n662 = call-dynamic "Read Text Font.vi"("error in (no error)"=w1275, "Control in"=w1265) -> ("error out"=w1274:errorcluster, "Font"=w1277:T1, "Control out"=w1278:refnum<class "Control.lvclass">)  [unwired: 7 out]
        n663 = call <userlib>:"Write INI Cluster__ogtk.vi"("error in (no error)"=w1274, "INI Fomatted Cluster"=w1277, "refnum"=w1289) -> ("error out"=w1287:errorcluster, "dup refnum"=w1288:T24)  [unwired: 1 in, 6 out]
        n664 = Bundle By Name(cluster=w1290, "Control"=w1278) -> (w1291:T20)
        n665 = call <vilib>:"Close Config Data.vi"("error in (no error)"=w1287, "refnum"=w1288) -> ("error out"=w1294:errorcluster)  [unwired: 1 in, 8 out]
        n666 = call <vilib>:"Add State(s) to Queue__jki_lib_state_machine.vi"("State(s) in (\"\")"=w1292) -> ("States Out"=w1293:string)  [unwired: 2 in, 12 out]
      }
      frame "Control: Set to Last State" {
        n667 = Unbundle By Name(w1335) -> ("Control"=w1334:refnum<class "Control.lvclass">, "last state"=w1327:T22, "user events"=w1325:T5)
        n668 = call-dynamic "Read Text Font.vi"("error in (no error)"=w1314, "Control in"=w1334) -> ("error out"=w1299:errorcluster, "Font"=w1308:T1)  [unwired: 8 out]
        n669 = Unbundle By Name(w1325) -> ("Icon (*.png)"=w1319:refnum<user-event>, "Action"=w1324:refnum<user-event>, "Orientations"=w1322:refnum<user-event>, "Font"=w1310:refnum<user-event>, "Control Text"=w1309:refnum<user-event>, "Style"=w1305:refnum<user-event>, "Text Color"=w1303:refnum<user-event>, "Scale Icon"=w1300:refnum<user-event>)
        n670 = Unbundle By Name(w1327) -> ("Action"=w1323:T2, "Orientations"=w1321:T3, "Icon (*.png)"=w1318:path, "Control Text"=w1307:string, "Style"=w1304:u16, "Text Color"=w1302:u32, "Scale"=w1298:dbl)  [unwired: 1 out]
        n671 = Generate User Event(user event=w1300, event data cluster=w1298, error in=w1299) -> (error out=w1301:errorcluster)  [unwired: 1 in, 1 out]
        n672 = Generate User Event(user event=w1303, event data cluster=w1302, error in=w1301) -> (error out=w1312:errorcluster)  [unwired: 1 in, 1 out]
        n673 = Generate User Event(user event=w1305, event data cluster=w1304, error in=w1312) -> (error out=w1306:errorcluster)  [unwired: 1 in, 1 out]
        n674 = Generate User Event(user event=w1309, event data cluster=w1307, error in=w1306) -> (error out=w1313:errorcluster)  [unwired: 1 in, 1 out]
        n675 = call-poly <userlib>:"File Exists__ogtk.vi"("file path"=w1318) -> ("exists"=w1333:bool)  [unwired: 6 in, 1 out]
        n676 = Empty String/Path?(string/path=w1318) -> (empty?=w1332:bool)
        n677 = Generate User Event(user event=w1310, event data cluster=w1308, error in=w1313) -> (error out=w1311:errorcluster)  [unwired: 1 in, 1 out]
        n678 = Generate User Event(user event=w1322, event data cluster=w1321, error in=w1311) -> (error out=w1317:errorcluster)  [unwired: 1 in, 1 out]
        n679 = Compound Arithmetic op=AND(w1333, invert w1332) -> (w1320:bool)
        n680 = Generate User Event(user event=w1324, event data cluster=w1323, error in=w1317) -> (error out=w1316:errorcluster)  [unwired: 1 in, 1 out]
        n681 = Select(t="", s=w1320, f="Control: Browse Icon") -> (s? t:f=w1329:string)
        n682 = case shown="True" w1320 {
          tunnel: w1319 -> [_ w1340]
          tunnel: w1318 -> [_ w1339]
          tunnel: w1316 -> [w1336 w1338]
          tunnel: [w1336 w1337] -> w1315
          frame False {
          }
          frame True {
            n683 = Generate User Event(user event=w1340, event data cluster=w1339, error in=w1338) -> (error out=w1337:errorcluster)  [unwired: 1 in, 1 out]
          }
        }
        n684 = call <vilib>:"Add State(s) to Queue__jki_lib_state_machine.vi"("State(s) in Front (\"\")"=w1329, "State(s) in (\"\")"=w1328) -> ("States Out"=w1326:string)  [unwired: 1 in, 12 out]
      }
      frame "Control: Browse Icon" {
        n685 = Unbundle By Name(w1347) -> ("Control"=w1348:refnum<class "Control.lvclass">)
        n686 = call <userlib>:"Current VIs Parent Directory__ogtk.vi"("Relative path (.)"=path "config.ini") -> ("Parent Directory (+ Relative)"=w1351:path)  [unwired: 4 out]
        n687 = call "Get Icon Source Path INI.vi"("error in"=w1342, "config.ini path"=w1351) -> ("error out"=w1343:errorcluster, "Icon source dir"=w1350:path, "config.ini path dup"=w1349:path)  [unwired: 1 in, 6 out]
        n688 = call "File Dialog2"("start path"=w1350, "prompt"="Select a single PNG file or choose a source directory for batch processing." ("pattern label"), "error in"=w1343, "pattern (all files)"="*.png", "pattern label"="PNG files") -> ("selected path"=w1353:path, "cancelled"=w1356:bool, "error out"=w1357:errorcluster)  [unwired: 2 in, 6 out]
        n689 = case shown="False" w1356 {
          tunnel: [w1376 w1381] -> w1345
          tunnel: w1348 -> [w1374 w1381]
          tunnel: w1357 -> [w1373 w1379]
          tunnel: [w1371 w1378] -> w1341
          tunnel: w1353 -> [w1365 _]
          tunnel: w1349 -> [w1368 _]
          tunnel: ["Preview" ("State(s) in Front (\"\")") "Error >> 7001" ("State(s) in Front (\"\")")] -> w1344
          frame False {
            n690 = local read "Same decal True/False"() -> (w1364:bool)
            n691 = call-poly <userlib>:"Strip Path__ogtk.vi"("path"=w1365) -> ("stripped path"=w1367:path, "name"=w1370:string)
            n692 = property on="Icon source" class="Path"("Value"=w1365) -> ()  [unwired: 2 in, 2 out]
            n693 = local read "TRUE Text"() -> (w1363:string)
            n694 = call-poly <userlib>:"Strip Path Extension__ogtk.vi"("path"=w1370) -> ("root"=w1369:string)  [unwired: 1 out]
            n695 = call-dynamic "Load Icon.vi"("error in (no error)"=w1373, "Icon path False"=w1365, "Control in"=w1374) -> ("error out"=w1372:errorcluster, "Control out"=w1375:refnum<class "Control.lvclass">)  [unwired: 1 in, 6 out]
            n696 = call-poly <userlib>:"To Proper Case__ogtk.vi"("string"=w1369) -> ("proper case string"=w1362:string)  [unwired: 4 out]
            n697 = local write "FALSE Text"(w1362) -> ()
            n698 = call "Set Icon Source Path INI.vi"("Icon source dir"=w1367, "config.ini path"=w1368) -> ()  [unwired: 1 in, 9 out]
            n699 = Select(t=w1362, s=w1364, f=w1363) -> (s? t:f=w1361:string)
            n700 = call-dynamic "Write Control Text.vi"("error in (no error)"=w1372, "True Text"=w1361, "False Text"=w1362, "Control in"=w1375) -> ("error out"=w1371:errorcluster, "Control out"=w1376:refnum<class "Control.lvclass">)  [unwired: 6 out]
          }
          frame True {
            n701 = Unbundle By Name(w1379) -> ("code"=w1380:i32)
            n702 = case shown="Default" w1380 {
              tunnel: [w1382 w1383] -> w1378
              tunnel: w1379 -> [w1382 w1384]
              frame Default {
              }
              frame 43 {
                n703 = call <vilib>:"Clear Errors.vi"("error in (no error)"=w1384) -> ("error out"=w1383:errorcluster)  [unwired: 6 out]
              }
            }
          }
        }
        n704 = Bundle By Name(cluster=w1347, "Control"=w1345) -> (w1346:T20)
        n705 = call <vilib>:"Add State(s) to Queue__jki_lib_state_machine.vi"("State(s) in Front (\"\")"=w1344, "State(s) in (\"\")"=w1360) -> ("States Out"=w1359:string)  [unwired: 1 in, 12 out]
      }
    }
  }
